vi "GESTIONE ALIMENTATORI.vi"(10 "Sub Panel alim1":refnum<vi>, 11 "Alimentatore":i32=1) -> ()   [LabVIEW 2019]
uses:
  TypeDef/Alimentatore.ctl
  Rampe e compensazioni/Comandi alimentatori.ctl
  TypeDef/Comandi_Alimentatore.ctl
  cDAQ_PLC Folder/cDAQ/SET SINGLE DO.ctl
  cDAQ_PLC Folder/cDAQ/DO List.ctl
  cDAQ_PLC Folder/cDAQ/SET SINGLE AO.ctl
  cDAQ_PLC Folder/cDAQ/AO List.ctl
  cDAQ_PLC Folder/cDAQ/SET ARRAY DO.ctl
  Stato alimentatore 1.vi
  Fine rampa sinus penta.vi
  Global_All_Data.vi
  Global FINE AVVIO.vi
  Global rapporto trasfo.vi
  Global dati targa SINUSPENTA.vi
panel:
  in  "Time Target (s)":dbl=1.0
  out "RPM":dbl
  out "Alimentatore selez":i32
  out "Iteration in Loop 1":i32
  out "Message":string
  in  "y 2":dbl=49.0 format="%#_13g"
  in  "y":dbl=5.0 format="%#_13g"
  out "Nome":string
  in  "SELEZIONA ALIMENTATORE":bool
  in  "indice alimentatore":i8
  out "Boolean":bool
  in  "Alimentatore":T1 {"Status ref"."RIF 2" scale=0.0..100.0; "Status ref"."RIF 1" scale=0.0..400.0}
  out "Alimentatore 1":T1 {"Status ref"."RIF 2" scale=0.0..100.0; "Status ref"."RIF 1" scale=0.0..100.0}
  in  "Salva alimentatori":bool
  in  "EXIT":bool
  out "EXIT":bool
  out "Comandi alimentatori":T2[](array[typedef])
  in  "Misure":T3
  in  "Array pannelli alimentatori":T4(array[cluster])
  in  "Array alimentatori":T5[](array[typedef]) {"Controllo Rif 2"."Precisione pid" format="%#_13g"; "Controllo Rif 2"."PID gains"."derivative time (Td, min)" format="%.3f"; "Controllo Rif 2"."PID gains"."integral time (Ti, min)" format="%.3f"; "Controllo Rif 2"."PID gains"."proportional gain (Kc)" format="%.3f"; "Controllo Rif 1"."Precisione pid" format="%#_13g"; "Controllo Rif 1"."PID gains"."derivative time (Td, min)" format="%.3f"; "Controllo Rif 1"."PID gains"."integral time (Ti, min)" format="%.3f"; "Controllo Rif 1"."PID gains"."proportional gain (Kc)" format="%.3f"}
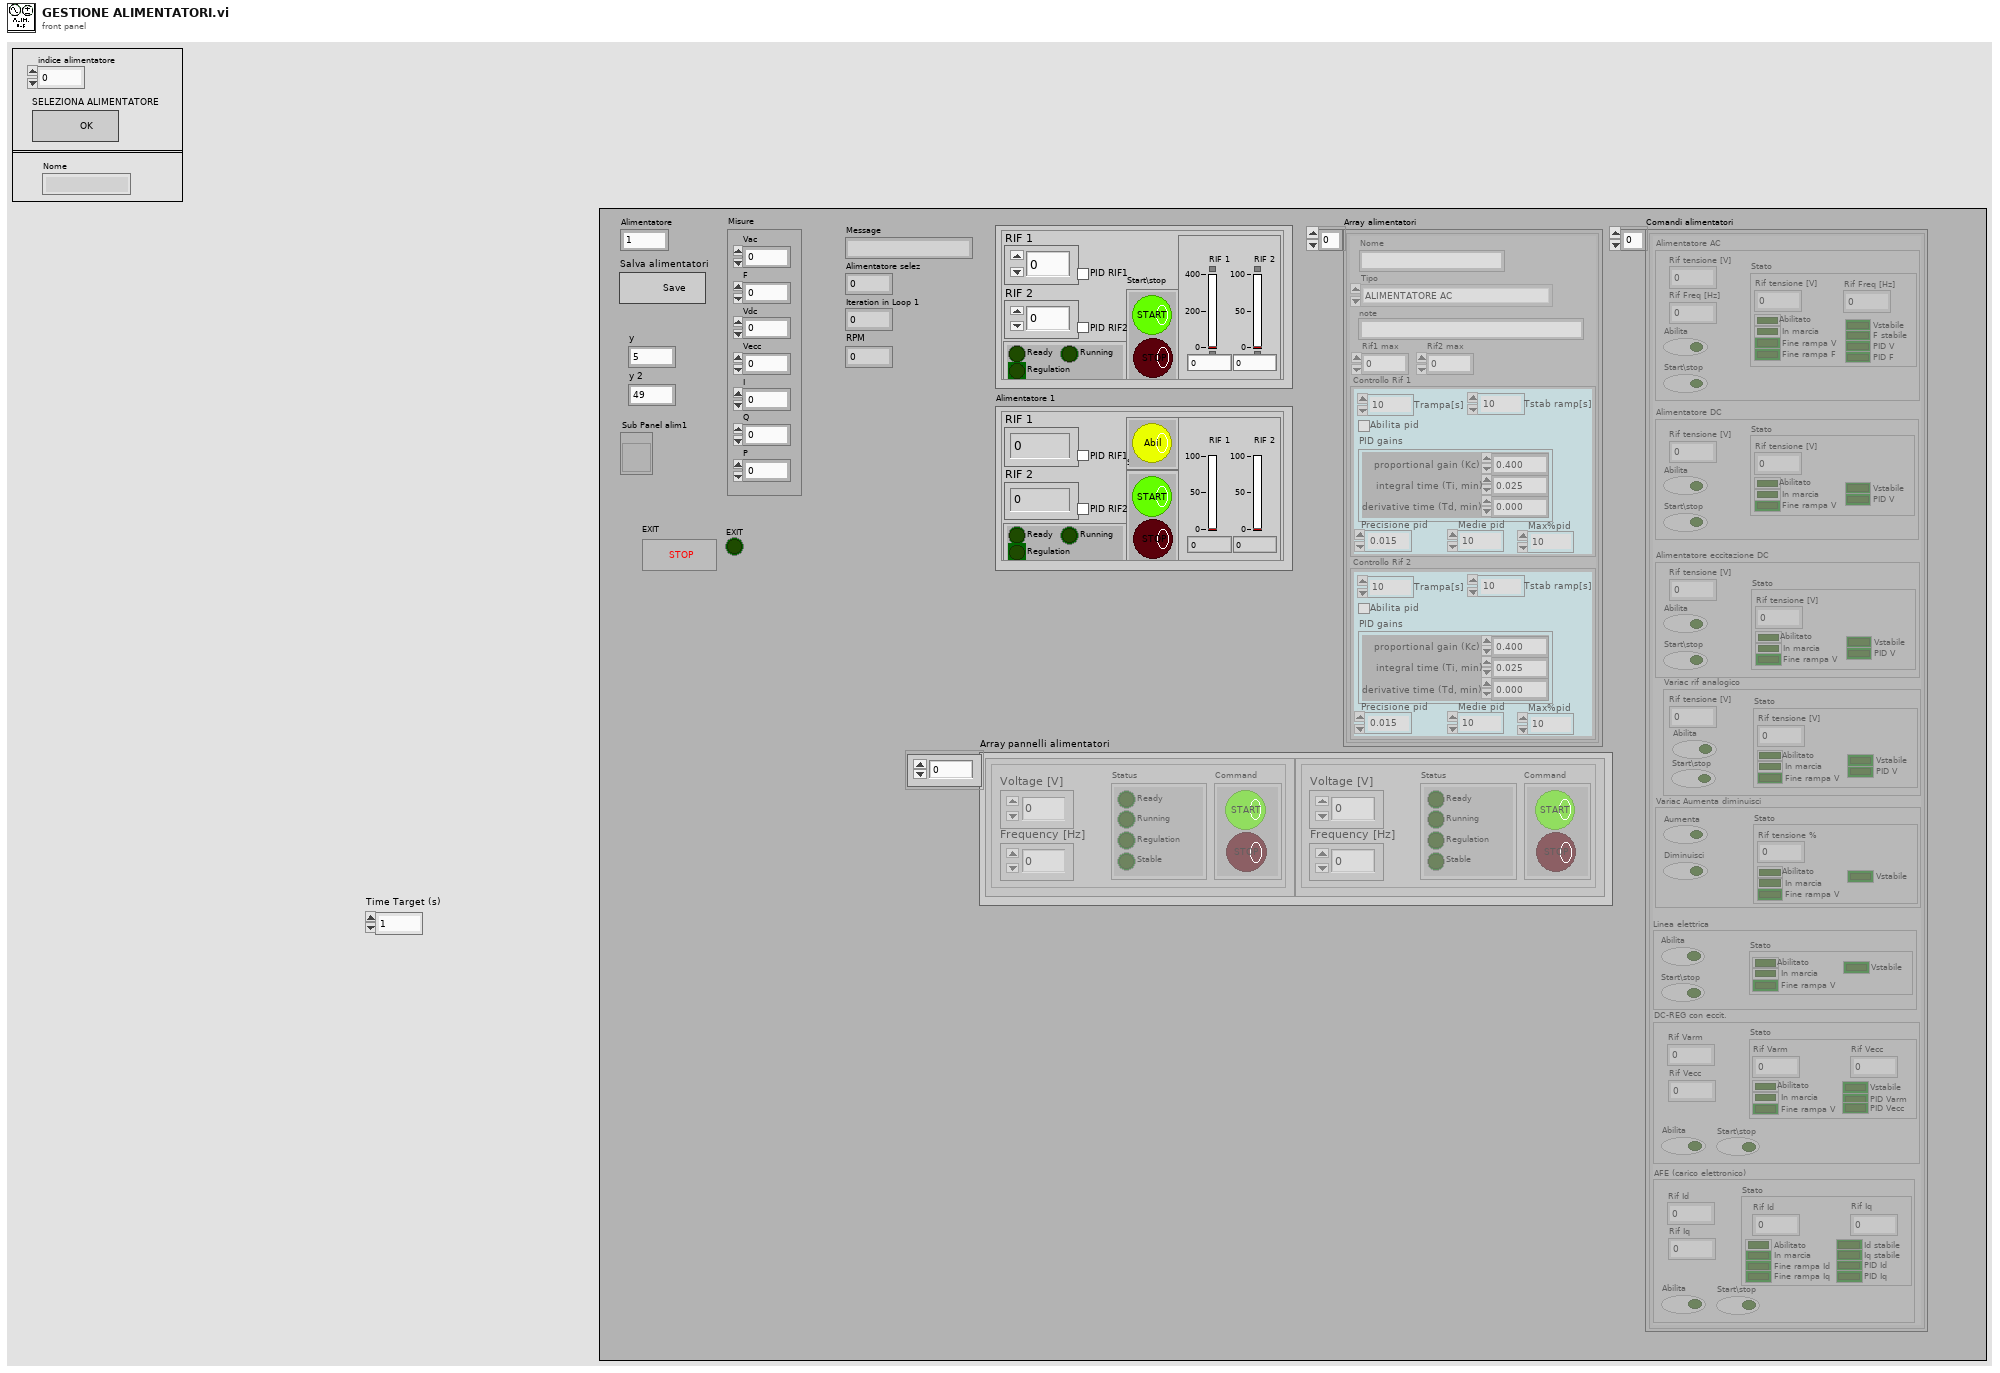
[diagram p1: front panel]
types:
  T1 = typedef "Comandi_Alimentatore.ctl" = cluster{"RIF 1":dbl, "RIF 2":dbl, "Status":cluster{"Ready":bool, "Running":bool, "Regulation":bool}, "Start\\stop":cluster{"Start":bool, "Stop":bool}, "PID RIF1":bool, "PID RIF2":bool, "Status ref":cluster{"RIF 1":dbl, "RIF 2":dbl}, "Abilita":cluster{"Abilita":bool}}
  T2 = typedef "Comandi alimentatori.ctl" = cluster{"Alimentatore AC":cluster{"Rif tensione [V]":dbl, "Rif Freq [Hz]":dbl, "Abilita":bool, "Start\\stop":bool, "Stato":cluster{"Rif tensione [V]":dbl, "Rif Freq [Hz]":dbl, "Abilitato":bool, "In marcia":bool, "Fine rampa V":bool, "Fine rampa F":bool, "Vstabile":bool, "F stabile":bool, "PID V":bool, "PID F":bool}}, "Alimentatore DC":cluster{"Rif tensione [V]":dbl, "Abilita":bool, "Start\\stop":bool, "Stato":cluster{"Rif tensione [V]":dbl, "Abilitato":bool, "In marcia":bool, "Fine rampa V":bool, "Vstabile":bool, "PID V":bool}}, "Variac rif analogico":cluster{"Rif tensione [V]":dbl, "Stato":cluster{"Rif tensione [V]":dbl, "Abilitato":bool, "In marcia":bool, "Fine rampa V":bool, "Vstabile":bool, "PID V":bool}, "Start\\stop":bool, "Abilita":bool}, "Variac Aumenta diminuisci":cluster{"Aumenta":bool, "Diminuisci":bool, "Stato":cluster{"Rif tensione %":dbl, "Abilitato":bool, "In marcia":bool, "Fine rampa V":bool, "Vstabile":bool}}, "Alimentatore eccitazione DC":cluster{"Rif tensione [V]":dbl, "Abilita":bool, "Start\\stop":bool, "Stato":cluster{"Rif tensione [V]":dbl, "Abilitato":bool, "In marcia":bool, "Fine rampa V":bool, "Vstabile":bool, "PID V":bool}}, "Linea elettrica":cluster{"Abilita":bool, "Start\\stop":bool, "Stato":cluster{"Abilitato":bool, "In marcia":bool, "Fine rampa V":bool, "Vstabile":bool}}, "DC-REG con eccit.":cluster{"Rif Varm":dbl, "Abilita":bool, "Start\\stop":bool, "Stato":cluster{"Rif Varm":dbl, "Abilitato":bool, "In marcia":bool, "Fine rampa V":bool, "Vstabile":bool, "PID Varm":bool, "Rif Vecc":dbl, "PID Vecc":bool}, "Rif Vecc":dbl}, "AFE (carico elettronico)":cluster{"Rif Id":dbl, "Abilita":bool, "Start\\stop":bool, "Stato":cluster{"Rif Id":dbl, "Rif Iq":dbl, "Abilitato":bool, "In marcia":bool, "Fine rampa Id":bool, "Fine rampa Iq":bool, "Id stabile":bool, "Iq stabile":bool, "PID Id":bool, "PID Iq":bool}, "Rif Iq":dbl}}
  T3 = cluster{"Vac":dbl, "F":dbl, "Vdc":dbl, "Vecc":dbl, "I":dbl, "Q":dbl, "P":dbl}
  T4 = cluster{"Voltage [V]":dbl, "Frequency [Hz]":dbl, "Status":cluster{"Ready":bool, "Running":bool, "Regulation":bool, "Stable":bool}, "Command":cluster{"Start":bool, "Stop":bool}}[]
  T5 = typedef "Alimentatore.ctl" = cluster{"Rif1 max":dbl, "Rif2 max":dbl, "Tipo":enum16{"ALIMENTATORE AC", "VARIAC AC rif analogico", "VARIAC AC aumenta diminuisci", "ALIMENTATORE DC", "ALIMENTATORE eccitazione DC", "LINEA ELETTRICA", "DCREG con eccitazione", "Carico elettronico AFE"}, "Nome":string, "Controllo Rif 1":cluster{"PID gains":cluster{"proportional gain (Kc)":dbl, "integral time (Ti, min)":dbl, "derivative time (Td, min)":dbl}, "Abilita pid":bool, "Precisione pid":dbl, "Medie pid":i32, "Trampa[s]":i32, "Tstab ramp[s]":i32, "Max%pid":i32}, "Controllo Rif 2":cluster{"PID gains":cluster{"proportional gain (Kc)":dbl, "integral time (Ti, min)":dbl, "derivative time (Td, min)":dbl}, "Abilita pid":bool, "Precisione pid":dbl, "Medie pid":i32, "Trampa[s]":i32, "Tstab ramp[s]":i32, "Max%pid":i32}, "note":string}
  T6 = cluster{"Message":string, "Message Data":variant}
  T7 = cluster{"RIF 1":dbl, "RIF 2":dbl, "Status":cluster{"Ready":bool, "Running":bool, "Regulation":bool, "Stable":bool}, "Command":cluster{"Start":bool, "Stop":bool}}
  T8 = enum16{"open", "replace", "create", "open or create", "replace or create", "replace or create with confirmation"}
  T9 = cluster{"RIF1":dbl, "RIF2":dbl, "Status":cluster{"Ready":bool, "Running":bool, "Regulation":bool, "Stable":bool}, "Command":cluster{"Start":bool, "Stop":bool}}[]
  T10 = cluster{"Voltage [V]":dbl, "Frequency [Hz]":dbl, "Status":cluster{"Ready":bool, "Running":bool, "Regulation":bool, "Stable":bool}, "Command":cluster{"Start":bool, "Stop":bool}}
  T11 = cluster{"RIF 1":dbl, "RIF 2":dbl, "Status":cluster{"Ready":bool, "Running":bool, "Regulation":bool, "Stable":bool}, "Command":cluster{"Start":bool, "Stop":bool}}[]
  T12 = cluster{"RIF1":dbl, "RIF2":dbl, "Status":cluster{"Ready":bool, "Running":bool, "Regulation":bool, "Stable":bool}, "Command":cluster{"Start":bool, "Stop":bool}}
  T13 = enum16{"ALIMENTATORE AC", "VARIAC AC rif analogico", "VARIAC AC aumenta diminuisci", "ALIMENTATORE DC", "ALIMENTATORE eccitazione DC", "LINEA ELETTRICA", "DCREG con eccitazione", "Carico elettronico AFE"}
  T14 = cluster{"PID gains":cluster{"proportional gain (Kc)":dbl, "integral time (Ti, min)":dbl, "derivative time (Td, min)":dbl}, "Abilita pid":bool, "Precisione pid":dbl, "Medie pid":i32, "Trampa[s]":i32, "Tstab ramp[s]":i32, "Max%pid":i32}
  T15 = cluster{"RIF 1":dbl, "RIF 2":dbl, "Abilitato":bool, "In marcia":bool, "Fine rampa RIF1":bool, "Fine rampa RIF2":bool, "Vstabile":bool, "F stabile":bool, "PID RIF1":bool, "PID RIF2":bool, "Alimentatore 1":T1}
  T16 = typedef "SET SINGLE DO.ctl" = cluster{"DO":T17, "Value":bool}
  T17 = typedef "DO List.ctl" = enum16{"OFF: ALL DO", "*ABILITA freno 1", "*ABILITA freno 2", "*ABILITA freno 3", "*START freno 1", "*START freno 2", "*START freno 3", "*STOP freno 1", "*STOP freno 3", "*STOP freno 2", "*Senso rot freno 1", "*Senso rot freno 2", "*Senso rot freno 3", "*Ctrl velocità freno 1", "*Ctrl velocità freno 2", "*Ctrl velocità freno 3", "*Ctrl coppia freno 1", "*Ctrl coppia freno 2", "*Ctrl coppia freno 3", "*ABILITA alimentatore 1", "*ABILITA alimentatore 2", "*ABILITA alimentatore 3", "*ABILITA alimentatore 4", "*START alimentatore 1", "*START alimentatore 2", "*START alimentatore 3", "*START alimentatore 4", "*STOP alimentatore 1", "*STOP alimentatore 2", "*STOP alimentatore 3", "*STOP alimentatore 4", "SENSO ROT alimentatore 1", "SENSO ROT alimentatore 2", "Abilita LEM 1000A", "Abilita LEM 300A", "Abilita sensori EXT WT", "B1 Seleziona linea 1", "B1 Seleziona linea 2", "B1 Seleziona linea 3", "B1 Seleziona linea 4", "B1 Seleziona linea 5", "B2 Seleziona linea 1", "B2 Seleziona linea 2", "B2 Seleziona linea 3", "B2 Seleziona linea 4", "B2 Seleziona linea 5", "*Reset allarmi", "*Start potenza AC", "*Stop potenza AC", "*Start potenza DC", "*Stop potenza DC", "*Start potenza DC eccit", "*Stop pontenza DC eccit", "Bypass res meter", "2nd canale res meter", "Enable res meter", "*Abilit teler ramo WT", "*Abil teler ramo princ Resit", "*Abil teler ramo 1 Resist", "*Abil teler ramo 2 Resist", "*Abil teler ramo 3 Resist", "*Abil cortocirc avvolgim", "*Controllo torsiometro B1", "*Controllo Torsiom B2", "*Scala torsiometro B1", "*Scala torsiometro B2", "*Collaudo in corso", "*Allarme presente", "Abilitazione elettroserratura", "Exit", "*Abilita collaudo", "*Abilita potenza trifase", "*Abilita potenza monofase", "*Abilita potenza DC", "*Abilita potenza DC eccit", "*Disabilita teleruttori potenza", "Set teleruttori prova a freddo", "Prova a freddo monofase", "Watchdog", "Forza DO PLC 3", "Forza DO PLC 2", "Forza DO PLC 1", "Forza DO cDAQ", "Scala 2000(T) 200(F) res meter", "Seleziona banco 1", "Seleziona banco 2", "Comando azionam in blocco", "Comando azionam reset", "Sensibilità freno 16 32 nm", "Reset Allarmi", "Carico res - Ramo 1", "Carico res - Ramo 2", "Carico res - Ramo 3", "Carico res - Ramo 4", "Carico res - Ramo 5", "Carico res - Ramo 6", "Carico res - Ramo 7", "Carico res - Ramo 8", "Carico res - Ramo 9", "Carico res - Ramo 10", "Carico res - Ramo 11", "Carico res - Start ventilatore", "Carico res - Stop ventilatore", "Abilita potenza solo freno", "Abilita AFE + freno trasc", "Abilita potenza carico resistivo", "Chiudi potenza AFE", "Apri potenza AFE", "Start AFE", "Config Banco2 TDE", "Misura diretto WT", "Ripristina centralina protezioni", "Abilita Scrittura Dati Keb", "Bench Selection(0-B1,1-B2)", "Select current mode", "Select torque mode", "Select speed mode", "Extenal alarm", "Enable Extenal program ", "Start ", "Stop", "Enable force mode", "Abilita linea 125 A", "Abilita linea 63 A", "Abilita linea 16 A", "Aum Tensione Variac", "Dim Tesnione Variac", "Abilita Ellecto Stractura", "Riprinto Emergenxe ", "Abilita Collaudo", "Disabilita Collaudo", "Abilita Ingresso Variac", "Abilita Uscita Variac", "Abilita ventilatore Variac"}
  T18 = typedef "SET SINGLE AO.ctl" = cluster{"AO":T19, "Value":dbl}
  T19 = typedef "AO List.ctl" = enum16{"OFF: ALL AO", "RIF VEL FRENO 1", "RIF VEL FRENO 2", "RIF VEL FRENO 3", "RIF COPPIA FRENO", "RIF COPPIA FRENO 1", "RIF COPPIA FRENO 2", "RIF COPPIA FRENO 3", "RIF CORRENTE FRENO 2", "RIF V ALIM 1", "RIF F ALIM 1", "RIF V ALIM 2", "RIF F ALIM 2", "RIF V ALIM 3", "RIF F ALIM 3", "RIF V ALIM 4", "RIF F ALIM 4", "FORZA AO PLC 3", "FORZA AO PLC 2", "FORZA AO PLC 1", "FORZA AO cDAQ", "Configura alimentatore keb", "Tempo rampa keb", "Condensatori", "Exit"}
  T20 = cluster{"Rif tensione [V]":dbl, "Rif Freq [Hz]":dbl, "Abilitato":bool, "In marcia":bool, "Fine rampa V":bool, "Fine rampa F":bool, "Vstabile":bool, "F stabile":bool, "PID V":bool, "PID F":bool, "Alimentatore 1":T1}
  T21 = typedef "SET ARRAY DO.ctl" = T16[]
  T22 = typedef "Cluster MISURE.ctl" = cluster{"MISURE NM":T23, "MISURE ALL":T24}
  T23 = typedef "MISURE NM.ctl" = cluster{"Banco":string, "Anno":string, "Numero":string, "Ntabella":string, "Misura":string, "Tipo Prova":string, "ProgressivoAcq":string, "Descrizione":string, "Data_ora":string, "t. acq [h:m:s]":string, "t. acq [min]":string, "t. acq [s]":string, "n [rpm]":string, "f [Hz]":string, "U1[V]":string, "U2 [V]":string, "U3 [V]":string, "U123_media [V]":string, "I1[A]":string, "I2[A]":string, "I3[A]":string, "I123_media [A]*I":string, "I_123_sbil [%]":string, "Ulin[V]":string, "Uc [V]":string, "Uaux [V]":string, "Ilin[A]*I":string, "Imar[A]":string, "Iaux[A]":string, "Uarm[V]":string, "Uecc[V]":string, "Iarm[A]*I":string, "Iecc[A]":string, "pf":string, "P1 [W]":string, "P1 [kW]":string, "Q [VAR]":string, "Q [kVAR]":string, "S [VA]":string, "S [kVA]":string, "P1arm[W]":string, "P1ecc[W]":string, "Parm[kW]":string, "P1ecc[kW]":string, "Cond[uF]":string, "P1_linea_6fili[W]":string, "P1_linea_6fili[kW]":string, "eta_gr_6fili [%]":string, "eta_inverter_6fili [%]":string, "pf_linea_6fili":string, "U4 [V]":string, "U5 [V]":string, "U6 [V]":string, "U456_media [V]":string, "I4 [A]":string, "I5 [A]":string, "I6 [A]":string, "I456_media [A]":string, "C [Nm]*C":string, "Cric [Nm]":string, "Cric\\Cnom":string, "Iric[A]":string, "Iric\\Inom":string, "P2_mecc [W]":string, "P2_mecc [kW]":string, "eta motore [%]":string, "Scorr[%]":string, "Tamb[°C]":string, "R1[ohm]":string, "R2[ohm]":string, "R3[ohm]":string, "Rmedia[ohm]":string, "DT_R1[°C]":string, "DT_R2[°C]":string, "DT_R3[°C]":string, "DT_media[°C]":string, "R_marcia[ohm]":string, "R_aux[ohm]":string, "DT_marcia[°C]":string, "DT_aux[°C]":string, "R_Arm[ohm]":string, "R_Ecc[ohm]":string, "DT_Arm[°C]":string, "DT_Ecc[°C]":string, "TambFreddo[°C]":string, "R1_freddo[ohm]":string, "R2_freddo[ohm]":string, "R3_freddo[ohm]":string, "Rmedia_freddo[ohm]":string, "R_Marcia_freddo[ohm]":string, "R_Aux_freddo[ohm]":string, "R_Arm_freddo[ohm]":string, "R_Ecc_freddo[ohm]":string, "TC1 [°C]":string, "TC2 [°C]":string, "TC3 [°C]":string, "TC4 [°C]":string, "TC5 [°C]":string, "TC6 [°C]":string, "TC7 [°C]":string, "TC8 [°C]":string, "PT1000_1[°C]":string, "PT1000_2[°C]":string, "PT1000_3[°C]":string, "Vdc eccitatrice[V]":string, "Idc eccitatrice[A]":string, "Vdc rotore[V]":string, "Idc rotore[A]":string, "Vac rotore[V]":string, "Iac rotore[V]":string, "V dinamo[V]":string, "Portata Q":string, "Pressione H":string, "U1'[V]":string, "U2'[V]":string, "U3'[V]":string, "I1'[A]":string, "I2'[A]":string, "I3'[A]":string, "U''R-N":string, "U''S-N":string, "U'' T-N":string, "U''R-S":string, "U''R-T":string, "U''S-T":string, "I1''[A]":string, "I2''[A]":string, "I3''[A]":string, "F''[Hz]":string, "P''[kW]":string, "CosFi''":string, "PT1000_4[°C]":string, "Scorta 3":string}
  T24 = typedef "Cluster misure ALL.ctl" = cluster{"Cluster READ NI":T25, "MISURE WT":T28, "Resistenze Resistomat":T29, "INTERFACCIA":T30, "FREDDO resistomat":cluster{"Res Ch1":dbl, "Res Ch2":dbl, "tAMB":dbl, "Res Ch3":dbl}, "STATO PLC 1":T35, "Res Ch2":dbl, "Res Ch2 2":dbl, "FREDDO res meter":cluster{"Res Ch1":dbl, "Res Ch2":dbl, "tAMB":dbl, "Res Ch3":dbl}, "Resistenze Res Meter":T29, "READ SINUS PENTA":T39, "STATO PLC 2":T40, "STATO PLC 3":T44, "DCREG":T48}
  T25 = typedef "Cluster NI.ctl" = cluster{"AI (0-10V)":cluster{"AI 0":dbl, "AI 1":dbl, "AI 2":dbl, "AI 3":dbl, "AI 4":dbl, "AI 5":dbl, "AI 6":dbl, "AI 7":dbl, "AI 8":dbl, "AI 9":dbl, "AI 10":dbl, "AI 11":dbl, "AI 12":dbl, "AI 13":dbl, "AI 14":dbl, "AI 15":dbl, "AI 16":dbl, "AI 17":dbl, "AI 18":dbl, "AI 19":dbl, "AI 20":dbl, "AI 21":dbl, "AI 22":dbl, "AI 23":dbl, "AI 24":dbl, "AI 25":dbl, "AI 26":dbl, "AI 27":dbl, "AI 28":dbl, "AI 29":dbl, "AI 30":dbl, "AI 31":dbl}, "StatoAO_Cdaq[0-10V]":cluster{"AO 1":dbl, "AO 2":dbl, "AO 3":dbl, "AO 4":dbl}, "Contatori [rpm]":cluster{"RPM 1":dbl, "RPM 2":dbl}, "StatoAO_Cdaq [4-20mA]":T26, "StatoDO_Cdaq":T27, "DI":cluster{"Scorta 0":bool, "Scorta 1":bool, "Scorta 2":bool, "Scorta 3":bool, "Scorta 4":bool, "Scorta 5":bool, "Scorta 6":bool, "Scorta 7":bool, "Scorta 8":bool, "Scorta 9":bool, "Scorta 10":bool, "Scorta 11":bool, "Scorta 12":bool, "Scorta 13":bool, "Scorta 14":bool, "Scorta 15":bool, "Scorta 16":bool, "Scorta 17":bool, "Scorta 18":bool, "Scorta 19":bool, "Scorta 20":bool, "Scorta 21":bool, "Scorta 22":bool, "Scorta 23":bool, "Scorta 24":bool, "Scorta 25":bool, "Scorta 26":bool, "Scorta 27":bool, "Scorta 28":bool, "Scorta 29":bool, "Scorta 30":bool, "Scorta 31":bool}, "AI (4-20mA)":cluster{"AI 0":dbl, "AI 1":dbl, "AI 2":dbl, "AI 3":dbl, "AI 4":dbl, "AI 5":dbl, "AI 6":dbl, "AI 7":dbl, "AI 8":dbl, "AI 9":dbl, "AI 10":dbl, "AI 11":dbl, "AI 12":dbl, "AI 13":dbl, "AI 14":dbl, "AI 15":dbl}, "TC [°C]":cluster{"tc 1":dbl, "tc 2":dbl, "tc 3":dbl, "tc 4":dbl}, "NI Read Values":cluster{"RPM":dbl, "Frequency":dbl, "Mod 1":cluster{"Torsiometro 1":dbl, "Torsiometro 2":dbl, "Strin Gauge 1":dbl, "Strin Gauge 2":dbl}, "Mod 2":cluster{"Termocoppia 1":dbl, "Termocoppia 2":dbl, "Termocoppia 3":dbl, "Termocoppia 4":dbl}, "Mod 3":cluster{"PT 100 1":dbl, "PT 100 2":dbl, "PT 100 3":dbl, "PT 100 4":dbl}}}
  T26 = typedef "StatoAO_cdaq.ctl" = cluster{"Cdaq_AO [0-10V] 0 for Torque":dbl, "Cdaq_AO [0-10V] 1":dbl, "Cdaq_AO [0-10V] 2":dbl, "Cdaq_AO [0-10V] 3":dbl}
  T27 = typedef "statoDO_Cdaq.ctl" = cluster{"Scorta 0":bool, "Scorta 1":bool, "Scorta 2":bool, "Scorta 3":bool, "Scorta 4":bool, "Scorta 5":bool, "Scorta 6":bool, "Scorta 7":bool, "Scorta 8":bool, "Scorta 9":bool, "Scorta 10":bool, "Scorta 11":bool, "Scorta 12":bool, "Scorta 13":bool, "Scorta 14":bool, "Scorta 15":bool, "Scorta 16":bool, "Scorta 17":bool, "Scorta 18":bool, "Scorta 19":bool, "Scorta 20":bool, "Scorta 21":bool, "Scorta 22":bool, "Scorta 23":bool, "Scorta 24":bool, "Scorta 25":bool, "Scorta 26":bool, "Scorta 27":bool, "Scorta 28":bool, "Scorta 29":bool, "Scorta 30":bool, "Scorta 31":bool}
  T28 = typedef "MISURE WT.ctl" = cluster{"URMS 1":dbl, "IRMS 1":dbl, "P 1":dbl, "S 1":dbl, "Q 1":dbl, "LAMBDA 1":dbl, "PHI 1":dbl, "F U 1":dbl, "F I 1":dbl, "NONE 1":dbl, "URMS 2":dbl, "IRMS 2":dbl, "P 2":dbl, "S 2":dbl, "Q 2":dbl, "LAMBDA 2":dbl, "PHI 2":dbl, "F U 2":dbl, "F I 2":dbl, "NONE 2":dbl, "URMS 3":dbl, "IRMS 3":dbl, "P 3":dbl, "S 3":dbl, "Q 3":dbl, "LAMBDA 3":dbl, "PHI 3":dbl, "F U 3":dbl, "F I 3":dbl, "NONE 3":dbl, "URMS SIGMA":dbl, "IRMS SIGMA":dbl, "P SIGMA":dbl, "S SIGMA":dbl, "Q SIGMA":dbl, "LAMBDA SIGMA":dbl, "PHI SIGMA":dbl, "F U SIGMA":dbl, "F I SIGMA":dbl, "NONE 4":dbl}
  T29 = typedef "ClusterRes.ctl" = cluster{"Res Ch1":dbl, "Res Ch2":dbl, "Res Ch3":dbl, "Tamb":dbl}
  T30 = typedef "INTERFACCIA.ctl" = cluster{"AI":cluster{"Portate":T31[], "Pressioni":T31[], "Coppie[Nm]":T31[], "Valvole prop %":T31[], "RPM":T31[], "Livelli":T31[], "Temperature":T31[], "Riferimenti %":T31[], "TENSIONI":T31[], "CORRENTI":T31[]}, "DI (logici)":cluster{"Start da pulsantiera":bool, "Stop da pulsantiera":bool, "Reset da pulsantiera":bool, "Sistema OK":bool, "Collaudo abilitato":bool, "Potenza trifase abilitata":bool, "Potenza monofase abilitata":bool, "Potenza DC abilitata":bool, "Potenza DC ECC abilitata":bool, "Start alimentazione AC":bool, "Start alimentazione DC":bool, "Start DC eccitazione":bool, "Teleruttore WT abilitato":bool, "Teleruttore Resistomat abilitato":bool, "Teleruttore corto fasi":bool, "Ramo 1 resistomat":bool, "Ramo 2 resistomat":bool, "Ramo 3 resistomat":bool, "B1 Scelta linea elettrica 1":bool, "B1 Scelta linea elettrica 2":bool, "B1 Scelta linea elettrica 3":bool, "B1 Scelta linea elettrica 4":bool, "B1 Scelta linea elettrica 5":bool, "B2 Scelta linea elettrica 1":bool, "B2 Scelta linea elettrica 2":bool, "B2 Scelta linea elettrica 3":bool, "B2 Scelta linea elettrica 4":bool, "B2 Scelta linea elettrica 5":bool, "Rotore bloccato 1":bool, "Rotore bloccato 2":bool, "FRENO 1 abilitato":bool, "FRENO 1 run":bool, "FRENO 1 senso rotaz":bool, "FRENO 1 ctrl velocità":bool, "FRENO 2 abilitato":bool, "FRENO 2 run":bool, "FRENO 2 senso rotaz":bool, "FRENO 2 ctrl velocità":bool, "ALIM 1 abilitato":bool, "ALIM 1 run":bool, "ALIM 2 abilitato":bool, "ALIM 2 run":bool, "ALIM 3 abilitato":bool, "ALIM 3 run":bool, "FRENO 1 ctrl coppia":bool, "FRENO 2 ctrl coppia":bool, "FRENO 3 ctrl coppia":bool, "DI (logici) aggiuntivi impianto":cluster{"Solo freno abilitato":bool, "Carico resistivo abilitato":bool, "AFE+freno abilitato":bool, "Protezioni chiuse":bool, "Start potenza AFE":bool, "AFE in marcia":bool}, "Misura corrente diretta WT":bool, "Misura corrente sens ext":bool, "Sens ext abilitati":bool}, "AO non scalati":T33, "AO scalati":T33, "DO (logici)":T34}
  T31 = typedef "ClusterMisura_e_Unità_INPUT.ctl" = cluster{"Misura":dbl, "UM":T32, "Descrizione":string}
  T32 = typedef "UnitàMisura.ctl" = enum16{"V", "mA", "Bar", "RPM", "m3/s", "m3/min", "m3/h", "l/s", "l/min", "in3/min", "ft3/min", "gpm", "igpm", "igph", "%", "°C", "m", "Nm", "A"}
  T33 = typedef "Lista AO sistema.ctl" = cluster{"FRENO1 rif vel":dbl, "FRENO1 rif Coppia":dbl, "FRENO2 rif vel":dbl, "FRENO2 rif Coppia":dbl, "ALIM1 rif V":dbl, "ALIM1 rif F":dbl, "ALIM2 rif V":dbl, "ALIM2 rif F":dbl, "ALIM3 rif V":dbl, "ALIM3 rif F":dbl, "Fnom keb":dbl, "Rpm nom keb":dbl, "Pnom keb":dbl, "Inom keb":dbl, "Vnom keb":dbl, "Rpm max keb":dbl, "Tempo rampa keb":dbl, "Tipo Mot keb":dbl, "FRENO  rif Coppia ":dbl, "FRENO  rif  Corrente":dbl}
  T34 = typedef "DOinterfaccia.ctl" = cluster{"Scelta banco 1":bool, "Scelta banco 2":bool, "Scelta banco 3":bool, "FRENO 1 abilita":bool, "FRENO 1 start":bool, "FRENO 1 senso rotaz":bool, "FRENO 1 ctrl velocità":bool, "FRENO 2 abilita":bool, "FRENO 2 start":bool, "FRENO 2 senso rotaz":bool, "FRENO 2 ctrl velocità":bool, "ALIM 1 abilita":bool, "ALIM 1 start":bool, "ALIM 2 abilita":bool, "ALIM 2 start":bool, "ALIM 3 abilita":bool, "ALIM 3 start":bool, "Abilita linea trifase":bool, "Abilita linea monofase":bool, "Abilita linea dc":bool, "Abilita linea dc eccit":bool, "B1 Linea elettrica 1":bool, "B1 Linea elettrica 2":bool, "B1 Linea elettrica 3":bool, "B1 Linea elettrica 4":bool, "B1 Linea elettrica 5":bool, "B2 Linea elettrica 1":bool, "B2 Linea elettrica 2":bool, "B2 Linea elettrica 3":bool, "B2 Linea elettrica 4":bool, "B2 Linea elettrica 5":bool, "Start potenza AC":bool, "Stop pontenza AC":bool, "Start potenza DC":bool, "Stop potenza DC":bool, "Start potenza eccitaz":bool, "Stop potenza eccitaz":bool, "Reset allarmi":bool, "watchdog":bool, "Scala torsiometro B1":bool, "Controllo torsiom B1":bool, "Scala torsiometro B2":bool, "Controllo torsiom B2":bool, "Teleruttore WT abilita":bool, "Teleruttore Resistomat abilita":bool, "Teleruttore corto fasi":bool, "Ramo 1 resistomat":bool, "Ramo 2 resistomat":bool, "Ramo 3 resistomat":bool, "Collaudo in corso":bool, "Allarme presente":bool, "Enable Res Meter":bool, "Bypass Res Meter":bool, "2nd canale Res Meter":bool, "Scala 200/2000 res meter":bool, "Taratura res meter":bool, "FRENO 1 ctrl coppia":bool, "FRENO 2 ctrl coppia":bool, "FRENO 3 ctrl coppia":bool, "Aggiuntivi impianto":cluster{"Senso rotazione alim 1":bool, "Senso rotazione alim 2":bool}, "ALIM 1 stop":bool, "ALIM 2 stop":bool, "ALIM 3 stop":bool, "FRENO 1 stop":bool, "FRENO 2 stop":bool, "FRENO 3 stop":bool, "B1 configurazione freno B":bool, "B2 configurazione freno B":bool, "Abilita scrittura KEB":bool, "Bench Selection (0-B1,1-B2)":bool, "Select current mode":bool, "Select torque mode":bool, "Select speed mode":bool, "Start":bool, "Stop":bool, "Block":bool, "Enable Force mode":bool, "Abilita linea 125 A":bool, "Abilita linea 63 A":bool, "Abilita linea 16 A":bool, "Aum Tensione Variac":bool, "Dim Tesnione Variac":bool, "Abilita ellectro stractura":bool, "Risprinito Emergence":bool, "Abilita collaudo":bool, "Disabilita collaudo":bool, "External Alaram":bool, "Enable external program":bool, "Reset":bool, "Abilita Ingresso Variac":bool, "Abilita Ventilatore Variac":bool, "Abilita Uscita Variac ":bool}
  T35 = typedef "STATO PLC 1.ctl" = cluster{"USCITE PLC":T36, "Stato DI_PLC":cluster{"Sistema OK":bool, "Rotore bloccato":bool, "Scorta 1":bool, "Prova diretto inverter":bool, "Prova con filtro LC":bool, "Teleruttore WT abilitato":bool, "Alim sinus penta abilitato":bool, "Alim sinus penta in marcia":bool, "Freno abilitato":bool, "Freno in marcia":bool, "Senso rotazione freno":bool, "Potenza abilitata":bool, "Scorta 3":bool, "Scorta 4":bool, "scorta 5":bool, "scorta 6":bool}, "AI plc":cluster{"Allarmi 1":dbl, "Allarmi 2":dbl, "Scorta 1":dbl, "Scorta 2":dbl, "RPM mot prova":dbl, "I mot prova":dbl, "RPM freno":dbl, "I freno":dbl, "Scorta 3":dbl, "Scorta 4":dbl}}
  T36 = typedef "Uscite PLC 1.ctl" = cluster{"AO (real) 2":cluster{"SCORTA 1":dbl, "SCORTA 2":dbl, "SCORTA 3":dbl, "SCORTA 4":dbl, "SCORTA 5":dbl, "SCORTA 6":dbl, "SCORTA 7":dbl, "SCORTA 8":dbl}, "statoAO_PLC out":T37, "DO (bit)":T38}
  T37 = typedef "statoAO_plc_1.ctl" = cluster{"Rif Lim coppia freno [%]":dbl, "Rif rpm freno [%]":dbl, "Rif coppia freno [%]":dbl, "Rif V alimentatore [%]":dbl, "Rif F alimentatore [%]":dbl}
  T38 = typedef "StatoDO_PLC_1.ctl" = cluster{"Scelta banco 1":bool, "Set dati motore freno 2":bool, "Diretto inverter":bool, "Filtro LC":bool, "Marcia ALIM (1s)":bool, "Marcia FRENO (1s)":bool, "Stop AFE (1s)":bool, "Stop freno (1s)":bool, "Reset allarmi":bool, "Watchdog":bool, "Senso rotazione":bool, "Abilita collaudo (1s)":bool, "Disabilita collaudo (1s)":bool, "Abilitazione ALIM":bool, "Abilitazione FRENO":bool, "Teleruttore WT":bool, "Senso rot motore prova":bool, "Scorta 7":bool, "Scorta 8":bool, "Scorta 9":bool, "Scorta 10":bool, "Scorta 11":bool, "Scorta 12":bool, "Scorta 13":bool}
  T39 = typedef "Parametri inverter letti.ctl" = cluster{"Menù Misure motore (M000-M030)":cluster{"Rif vel a regime (int)":u16, "Rif vel a regime (dec)":u16, "Rif vel dopo rampe (int)":u16, "Rif vel dopo rampe (dec)":u16, "RPM motore (int)":u16, "RPM motore (dec)":u16, "FREQout inverter":u16, "Rif coppia a regime(Nm)":u16, "Richiesta di coppia (Nm)":u16, "Coppia generata dal motore(Nm)":u16, "Rif coppia a regime(%)":u16, "Richiesta di coppia (%)":u16, "Coppia generata dal motore(%)":u16, "Coppia max richiesta prima delle rampe(Nm)":u16, "Coppia max richiesta dopo le rampe(Nm)":u16, "Limite di velocità prima delle rampe":u16, "Limite di velocità dopo le rampe":u16, "Coppia max richiesta prima delle rampe(%)":u16, "Coppia max richiesta dopo le rampe(%)":u16, "Rif di flusso":u16, "Corrente di uscita":u16, "Capacità termica del motore":u16, "Tensione di uscita":u16, "Potenza di uscita":u16, "Energia consumata (LSword)":u16, "Energia consumata (MSword)":u16, "Tensione bus DC":u16, "Tensione di rete":u16}, "Menù regolatore PID (M018-M024)":cluster{"Rif PID a regime(%)":u16, "Rif pid dopo rampe(%)":u16, "Retroazione del pid(%)":u16, "Errore del pid(%)":u16, "uscita del pid(%)":u16, "Rif del pid dopo le rampe":u16, "Retroazione del pid":u16}, "Menù ingressi digitali (M031-M036)":cluster{"Ingressi digitali ritardati":u16, "Ingressi digitali istantanei":u16, "Moresettiera comando loc":u16, "Morsett comando da seriale":u16, "Morsett comando bus di campo":u16, "Ing dig ausiliari da morsettiera":u16, "Ing dig ausiliari da seriale":u16}, "Menù riferimenti (M037-M051)":cluster{"Rif analog est REF":u16, "Rif analog est AIN1":u16, "Rif analog est AIN2":u16, "Rif analog est XAIN4":u16, "Rif analog est XAIN5":u16, "Rif velocità da seriale(int)":u16, "Rif velocità bus di campo(int)":u16, "Rif coppia da seriale":u16, "Rif coppia bus di campo":u16, "Rif del PID da seriale":u16, "Rif del PID da bus di campo":u16, "Retroazione del PID da seriale":u16, "Retroazione del PIDda bus di campo":u16, "Rif da encoder":u16, "Rif in frequenza":u16, "Rif velocità da seriale(dec)":u16, "Rif velocità bus di campo(dec)":u16}, "Menù rampe (P009-P033)":cluster{"Tempo di dec rampa di vel 1":u16, "Tempo di acc rampa di vel 2":u16, "Tempo di dec rampa di vel 2":u16, "Tempo di acc rampa di vel 1":u16, "Unità di mis tempi rampe vel 1/2":u16, "Tempo di acc rampa di vel 3":u16, "Tempo di dec rampa di vel 3":u16, "Tempo di acc rampa di vel 4":u16, "Tempo di dec rampa di vel 4":u16, "Unità di mis tempi rampe vel 3/4":u16, "Selettore arrottondam rampe":u16, "Tempo di arrotond iniz rampa acc":u16, "Tempo di arrotond finale rampa acc":u16, "Tempo di arrotond iniz rampa dec":u16, "Tempo di rampa di salita rif coppia":u16, "Tempo di rampa di discesa rif coppia":u16, "Unità di misura rampa coppia":u16, "Tempo rampa acc marcia jog":u16, "Tempo rampa dec marcia jog":u16, "Reset acc ai cambi pendenza":u16, "rampa di acc in fire mode":u16, "rampa di dec in fire mode":u16, "Tempo di arrotond finale rampa dec":u16}, "Menù controllo motore(C008-C128)":cluster{"Numero motori configurati":u16, "Tipo algoritmo di controllo Mot1":u16, "Tipo rif Mot1":u16, "Tensione nominale rete":u16, "Retroaz di vel da encoder Mot1":u16, "Tipo curva V/f Mot1":u16, "Rotazione delle fasi Mot1":u16, "Freq nominale del motore Mot1":u16, "RPM nominali del motore Mot1":u16, "Potenza nominale del motore Mot1":u16, "Corrente nominale del motore Mot1":u16, "Tensione nominale del motore mot1":u16, "Potenza a vuoto del motore Mot1":u16, "Corrente a vuoto del motore Mot1":u16, "Resistenza statorica del motore Mot1":u16, "Induttanza di dispersione Mot1":u16, "Induttanza mutua motore":u16, "Costante di tempo rotorica":u16, "Costante di tempo filtro pb":u16, "Velocità minima motore":u16, "Velocità massima motore":u16}, "Menù configurazione PID":cluster{"Selezione riferimento n.1":u16, "Selezione retroazione n.1":u16, "Modalità di fuzionamento PID":u16, "Termine derivativo calcolato su err o mis":u16, "Proporz moltiplica deriv e integrale":u16, "Azione del PID":u16}, "ID":dbl, "Menù uscite digitali":cluster{"MDO4 Inverter pronto":u16}, "Fcarrier":cluster{"Fcarrier Min (Hz)":u16, "Fcarrier Max (Hz)":u16}, "stato inverter M089":dbl, "Riferimenti":cluster{"Rif tensione":u16, "Rif velocità":u16}, "Comunicazione":bool, "Modalità stop":dbl}
  T40 = typedef "STATO PLC 2.ctl" = cluster{"USCITE PLC":T41, "Stato DI_PLC":cluster{"Sistema ok":bool, "Relè Resistomat abilitato":bool, "Freno abilitato":bool, "Freno in marcia":bool, "scorta b":bool, "scorta a":bool, "scorta 1":bool, "scorta 2":bool, "scorta 3":bool, "scorta 4":bool, "Scorta 5":bool, "Scorta 6":bool, "Scorta 7":bool, "Scorta 8":bool, "Scorta 9":bool, "Scorta 10":bool}, "AI plc":cluster{"Allarmi 1":dbl, "Allarmi 2":dbl, "TC 1":dbl, "TC 2":dbl, "TC 3":dbl, "TC 4":dbl, "TC 5":dbl, "TC 6":dbl, "TC 7":dbl, "TC 8":dbl, "PT1000 1":dbl, "PT1000 2":dbl, "PT1000 3":dbl, "PT1000 4":dbl}}
  T41 = typedef "Uscite PLC 2.ctl" = cluster{"AO (real) 2":cluster{"SCORTA 1":dbl, "SCORTA 2":dbl, "SCORTA 3":dbl, "SCORTA 4":dbl, "SCORTA 5":dbl, "SCORTA 6":dbl, "SCORTA 7":dbl, "SCORTA 8":dbl}, "statoAO_PLC out":T42, "DO (bit)":T43}
  T42 = typedef "statoAO_plc_2.ctl" = cluster{"Condensatori":dbl, "Scorta 1":dbl, "Scorta 2":dbl}
  T43 = typedef "StatoDO_PLC_2.ctl" = cluster{"Relè misura resistomat":bool, "Misura res ramo 1":bool, "Misura res ramo 2":bool, "Misura res ramo 3":bool, "Scelta banco 2":bool, "Scala Torsiometro":bool, "Ctrl torsiometro":bool, "Select current mode":bool, "Select Torque mode":bool, "Select speed mode":bool, "Watchdog":bool, "Scorta":bool, "Scorta 2":bool, "Scorta 3":bool, "Scorta 4":bool, "Scorta 5":bool, "Bench selection":bool, "External alarm":bool, "Enable external program":bool, "Reset allarmi":bool, "Start":bool, "Stop":bool, "Block":bool, "Scorta 6":bool}
  T44 = typedef "STATO PLC 3.ctl" = cluster{"USCITE PLC":T45, "Stato DI_PLC":cluster{"Sistema OK":bool, "Rotore bloccato":bool, "Filtro LC":bool, "Bypass Filtro LC":bool, "Scelta Trasformatore":bool, "Scelta Bypass trasformatore":bool, "Teleruttore wt abilitato":bool, "Alimentatore abilitato":bool, "Alimentatore in marcia":bool, "Scorta 1":bool, "Scorta 2":bool, "Scorta 3":bool, "Potenza abilitata":bool, "Alimentatore in allarme":bool, "Scorta 4":bool, "Conferma dati KEB":bool, "Scorta 5":bool, "Warning Inverter Alimentatore":bool, "Variac Abilitato":bool, "Linea 125 A abilitata":bool, "Linea 63 A abilitata":bool, "Linea 16 A abilitata":bool, "Scorta 6":bool, "Enable force mode":bool}, "AI plc":cluster{"Allarmi 1":dbl, "Allarmi 2":dbl, "RPM motore prova":dbl, "Corrente motore prova":dbl, "RPM freno":dbl, "Corrente freno":dbl, "Tipo motore keb":dbl, "I nom keb":dbl, "RPM nom keb":dbl, "V nom keb":dbl, "F nom keb":dbl, "T rampa keb":dbl, "scorta":dbl, "Scorta 2":dbl}}
  T45 = typedef "Uscite PLC 3.ctl" = cluster{"AO (real) 2":cluster{"SCORTA 1":dbl, "SCORTA 2":dbl, "SCORTA 3":dbl, "SCORTA 4":dbl, "SCORTA 5":dbl, "SCORTA 6":dbl, "SCORTA 7":dbl, "SCORTA 8":dbl}, "statoAO_PLC out":T46, "DO (bit)":T47}
  T46 = typedef "statoAO_plc_3.ctl" = cluster{"Rif velocità alimentatore":dbl, "Scorta":dbl, "Tipo Motore  keb":dbl, "I nom keb":dbl, "RPM nom keb":dbl, "V nom keb":dbl, "F nom keb":dbl, "t rampa keb":dbl}
  T47 = typedef "StatoDO_PLC_3.ctl" = cluster{"Select linea Inverter":bool, "Abilita sense wattmetro":bool, "Bypass filtro LC":bool, "Filtro LC":bool, "Bypass trasformatore":bool, "Trasformatore":bool, "Abilita uscite variac":bool, "Abilita linea 125 A":bool, "Abilita linea 63 A":bool, "Abilita linea 16 A":bool, "Abilita Scrittura Dati Keb":bool, "Abilita alimentatore":bool, "Marcia alimentatore (1s)":bool, "Stop alimentatore (1s)":bool, "Senso rot mot prova":bool, "Watchdog":bool, "Aumenta tensione variac":bool, "Diminuisci tensione variac ":bool, "Blocco elettroserrature":bool, "Ripristino emergence":bool, "Abilita ingresso variac":bool, "Abilita ventilatore variac":bool, "Reset Allarm":bool, "Scorta 1":bool, "Scorta 2":bool, "Scorta 3":bool, "Scorta 4":bool, "Scorta 5":bool, "Scorta 6":bool, "Scorta 7":bool, "Scorta 8":bool, "Scorta 9":bool, "Abilita collaudo":bool, "Disabilita collaudo ":bool, "Scorta 10":bool, "Scorta 11":bool, "Scorta 12":bool, "Scorta 13":bool, "Scorta 14":bool, "Scorta 15":bool}
  T48 = typedef "Parametri DCREG letti.ctl" = cluster{"Parametri di misura":cluster{"M000":dbl, "M001":dbl, "M002":dbl, "M003":dbl, "M004":dbl, "M005":dbl, "M006":dbl, "M007":dbl, "M008":dbl, "M009":dbl, "M010":dbl, "M011":dbl, "M012":dbl, "M013":dbl, "M014":dbl, "M015":dbl, "M016":dbl, "M017":dbl, "M018":dbl, "M019":dbl, "M020":dbl, "M021":dbl, "M022":dbl, "M023":dbl, "M024":dbl, "M025":dbl, "M026":dbl, "M027":dbl, "M028":dbl, "M029":dbl, "M030":dbl, "M031":dbl}, "Parametri di programmazione":cluster{"P000":dbl, "P001":dbl, "P002":dbl, "P003":dbl, "P004":dbl, "P005":dbl, "P006":dbl, "P010":dbl, "P011":dbl, "P012":dbl, "P013":dbl, "P014":dbl, "P015":dbl, "P016":dbl, "P030":dbl, "P031":dbl, "P032":dbl, "P033":dbl, "P034":dbl, "P035":dbl, "P036":dbl, "P037":dbl, "P038":dbl, "P039":dbl, "P040":dbl, "P050":dbl, "P051":dbl, "P052":dbl, "P053":dbl, "P054":dbl, "P055":dbl, "P056":dbl, "P057":dbl, "P058":dbl, "P059":dbl, "P060":dbl, "P061":dbl, "P062":dbl, "P070":dbl, "P071":dbl, "P073":dbl, "P074":dbl, "P076":dbl, "P077":dbl, "P079":dbl, "P080":dbl, "P082":dbl, "P083":dbl, "P084":dbl, "P085":dbl, "P086":dbl, "P087":dbl, "P088":dbl, "P100":dbl, "P101":dbl, "P102":dbl, "P103":dbl, "P104":dbl, "P110":dbl, "P111":dbl, "P120":dbl, "P121":dbl, "P122":dbl, "P123":dbl, "P124":dbl, "P125":dbl, "P126":dbl, "P127":dbl, "P128":dbl, "P129":dbl, "P130":dbl, "P131":dbl, "P132":dbl, "P133":dbl, "P134":dbl, "P150":dbl, "P151":dbl, "P152":dbl, "P153":dbl, "P154":dbl, "P155":dbl, "P156":dbl, "P157":dbl, "P158":dbl, "P170":dbl, "P171":dbl, "P172":dbl, "P173":dbl, "P174":dbl, "P175":dbl, "P176":dbl, "P177":dbl, "P178":dbl, "P179":dbl, "P180":dbl, "P181":dbl, "P182":dbl, "P183":dbl, "P184":dbl, "P185":dbl, "P186":dbl, "P187":dbl, "P188":dbl, "P189":dbl, "P190":dbl, "P191":dbl, "P192":dbl, "P193":dbl, "P194":dbl, "P195":dbl, "P196":dbl, "P197":dbl, "P198":dbl, "P199":dbl, "P211":dbl, "P212":dbl, "P213":dbl, "P214":dbl, "P215":dbl, "P216":dbl, "P217":dbl, "P221":dbl, "P222":dbl, "P223":dbl, "P224":dbl, "P230":dbl, "P231":dbl, "P240":dbl, "P250":dbl, "P251":dbl}, "Parametri di configurazione":cluster{"C000":dbl, "C001":dbl, "C002":dbl, "C010":dbl, "C011":dbl, "C012":dbl, "C014":dbl, "C015":dbl, "C016":dbl, "C017":dbl, "C018":dbl, "C030":dbl, "C050":dbl, "C051":dbl, "C052":dbl, "C060":dbl, "C061":dbl, "C062":dbl, "C063":dbl, "C070":dbl, "C072":dbl, "C074":dbl, "C090":dbl, "C091":dbl, "C092":dbl, "C093":dbl, "C094":dbl, "C100":dbl, "C101":dbl, "C102":dbl, "C103":dbl, "C105":dbl, "C106":dbl, "C107":dbl, "C108":dbl, "C110":dbl, "C111":dbl, "C112":dbl, "C120":dbl, "C121":dbl, "C122":dbl, "C130":dbl, "C131":dbl, "C132":dbl, "C133":dbl, "C134":dbl, "C135":dbl, "C141":dbl, "C142":dbl, "C143":dbl, "C150":dbl, "C151":dbl, "C153":dbl, "C154":dbl, "C155":dbl, "C156":dbl, "C157":dbl, "C158":dbl, "C159":dbl, "C160":dbl, "C161":dbl, "C162":dbl, "C163":dbl, "C164":dbl, "C165":dbl, "C170":dbl}, "Codice allarme":dbl, "Comunicazione":bool}
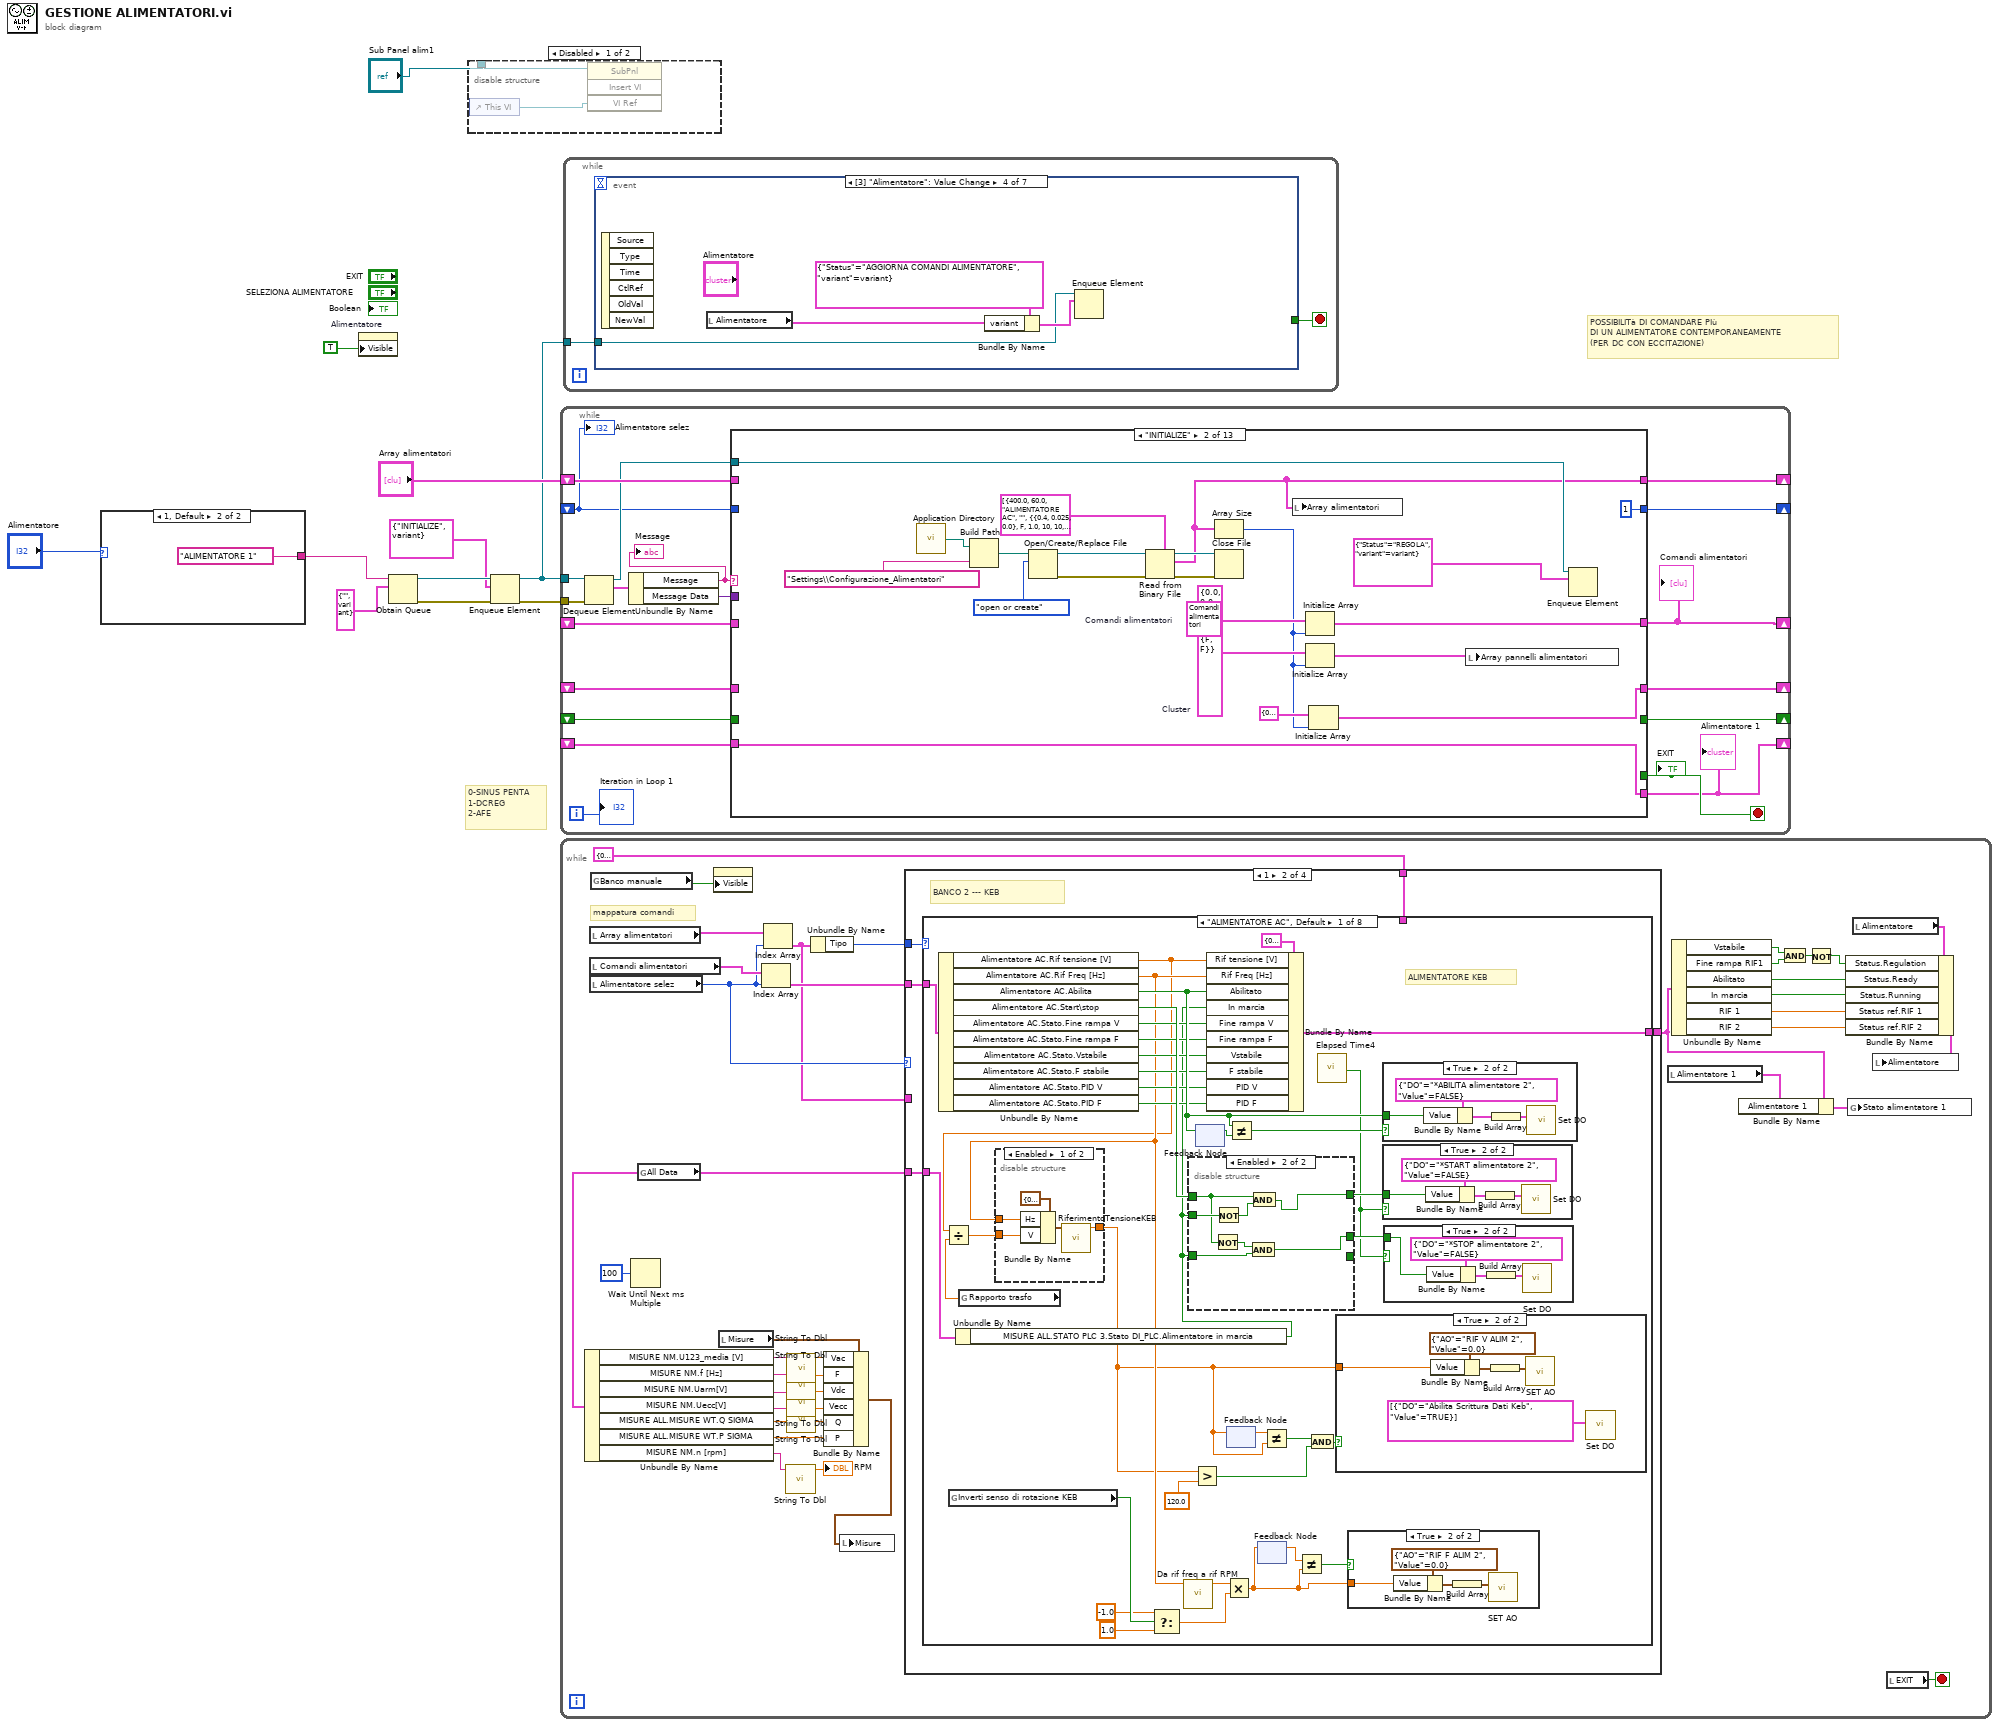
[diagram p0: block diagram]
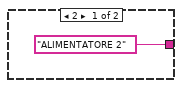
[diagram p3: hidden frame]
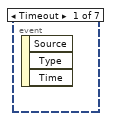
[diagram p4: hidden frame]
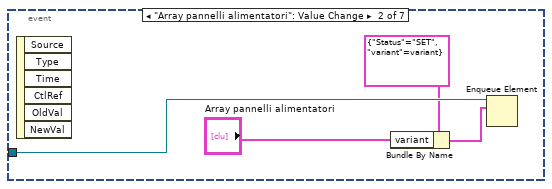
[diagram p5: hidden frame]
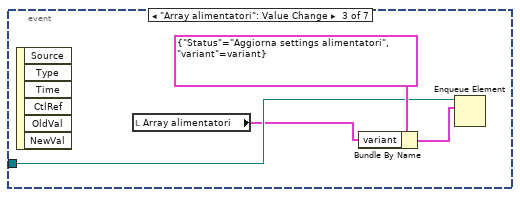
[diagram p6: hidden frame]
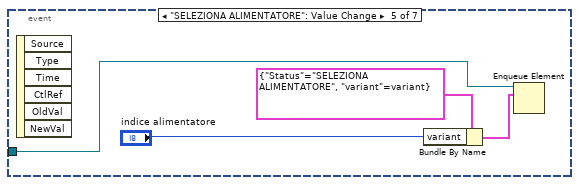
[diagram p7: hidden frame]
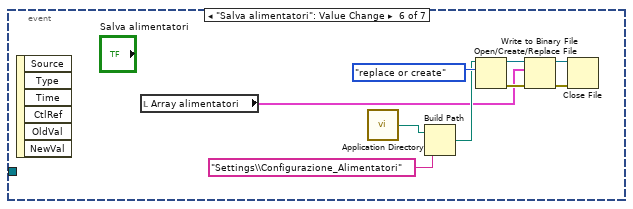
[diagram p8: hidden frame]
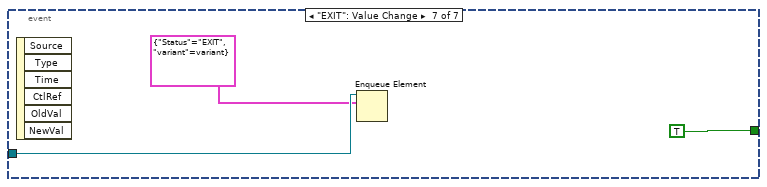
[diagram p9: hidden frame]
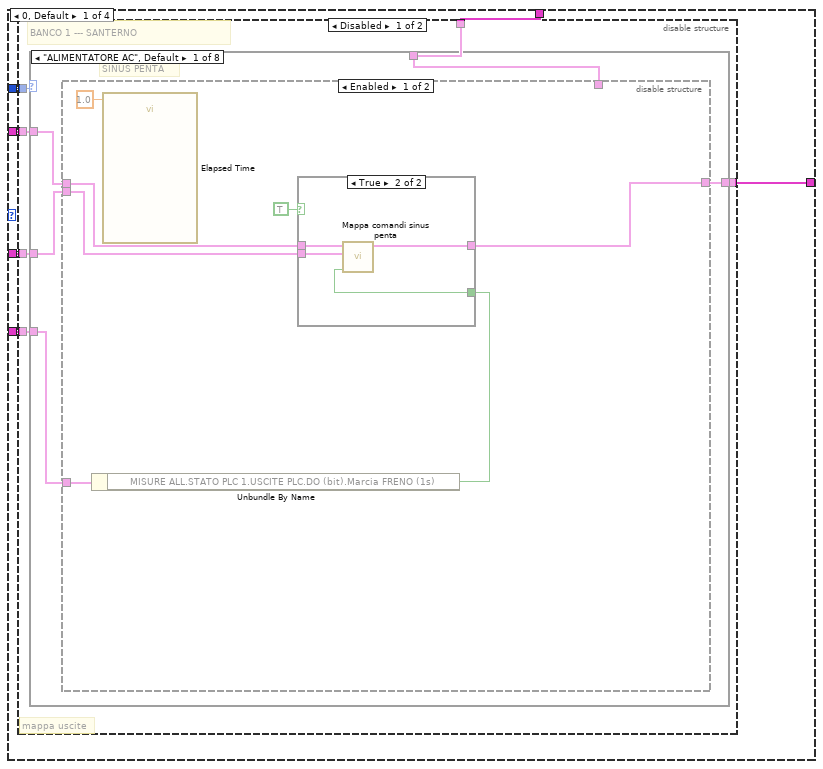
[diagram p10: hidden frame]
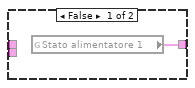
[diagram p11: hidden frame]
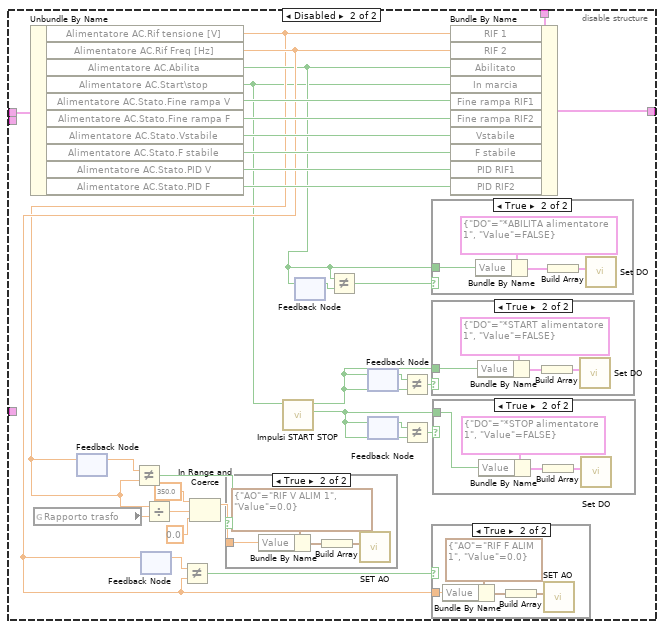
[diagram p12: hidden frame]
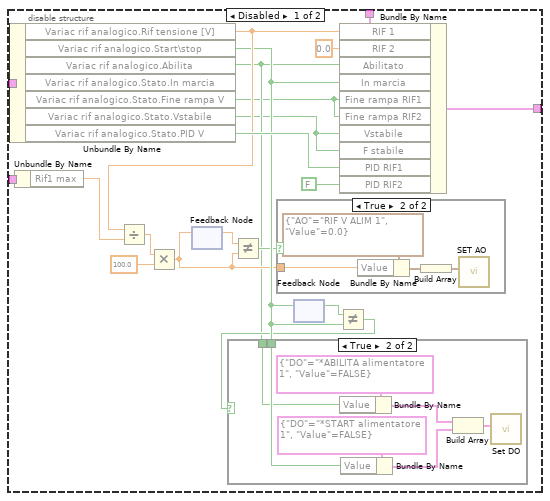
[diagram p19: hidden frame]
diagram:
  # "0-SINUS PENTA\n1-DCREG\n2-AFE"
  # "POSSIBILITà DI COMANDARE PIù\nDI UN ALIMENTATORE CONTEMPORANEAMENTE\n(PER DC CON ECCITAZIONE)"
  n1 = case shown="1, Default" "Alimentatore" {
    tunnel: ["ALIMENTATORE 2" ("name (unnamed)") "ALIMENTATORE 1" ("name (unnamed)")] -> w9
    frame 2 {
    }
    frame 1, Default {
    }
  }
  n2 = property on="Alimentatore" class="Clust (strict)"("Visible"=TRUE) -> ()  [unwired: 2 in, 2 out]
  n3 = Obtain Queue(name (unnamed)=w9, element data type=T6 {"Message"="", "Message Data"=variant} ("Message Cluster")) -> (queue out=w10:refnum<queue>, error out=w11:errorcluster)  [unwired: 3 in, 1 out]
  n4 = disable-structure shown="Disabled" {
    disable-tunnel: "Sub Panel alim1" -> [w15 _]
    frame Disabled {
      n5 = control-ref of="This VI"() -> (w14:refnum<vi>)
      n6 = invoke class="SubPnl" method="Insert VI"(reference=w15, "VI Ref"=w14) -> ()  [unwired: 2 in, 4 out]
    }
    frame Enabled {
    }
  }
  n7 = Enqueue Element(queue=w10, element=cluster{"Status":string, "variant":variant} {"Status"="INITIALIZE", "variant"=variant}, error in (no error)=w11) -> (queue out=w4:refnum<queue>, error out=w5:errorcluster)  [unwired: 1 in, 1 out]
  n8 = while {
    tunnel: w4 -> [w34]
    shift-right: [w30] -> _
    shift-left: "Array alimentatori" -> [w31]
    tunnel: w5 -> [w29]
    shift-right: [w17] -> _
    shift-left: _ -> [w28]
    shift-right: [w26] -> _
    shift-left: _ -> [w25]
    shift-right: [w24] -> _
    shift-left: _ -> [w23]
    shift-right: [w20] -> _
    shift-left: _ -> [w19]
    shift-right: [w16] -> _
    shift-left: _ -> [w18]
    i -> [w21]
    stop <- w27 stop-if-true
    n9 = Dequeue Element(queue=w34, error in (no error)=w29) -> (queue out=w22:refnum<queue>, element=w35:T6)  [unwired: 1 in, 2 out]
    n10 = Unbundle By Name(w35) -> ("Message"=w33:string, "Message Data"=w32:variant)
    "Message" <- w33
    n11 = case shown="\"INITIALIZE\"" w33 {
      tunnel: w32 -> [_ _ w84 w100 _ _ w286 w300 _ _ _ _ _]
      tunnel: w31 -> [w40 _ w81 w97 w105 w109 _ w297 w308 w342 w376 w408 w438]
      tunnel: [w40 w46 w79 w97 w105 w109 w284 w297 w308 w342 w376 w408 w438] -> w30
      tunnel: [w39 w60 w65 w96 w104 w123 w290 w296 w310 w344 w378 w410 w437] -> w17
      tunnel: w28 -> [w39 _ w65 w96 w104 w124 w290 w296 w312 w346 w380 w412 w437]
      tunnel: [_ _ _ _ _ _ _ _ _ _ _ _ w433] -> w27
      tunnel: [w38 w43 w73 w95 w103 w120 w289 w295 w309 w343 w377 w409 w436] -> w26
      tunnel: w25 -> [w38 _ w74 w95 w103 w120 w289 _ w309 w343 w377 w409 w436]
      tunnel: [_ _ TRUE w93 _ FALSE _ TRUE w311 w345 w379 w411 _] -> w24
      tunnel: w23 -> [_ _ _ w93 _ w121 _ _ w311 w345 w379 w411 _]
      tunnel: w22 -> [_ w59 w66 _ _ w118 _ w293 _ _ _ _ _]
      tunnel: [w36 w42 w63 w94 w101 w108 w288 w291 w302 w336 w370 w402 w434] -> w20
      tunnel: w19 -> [w36 w42 _ w94 w101 w108 w288 w291 w302 w336 w370 w402 w434]
      tunnel: [w37 1 w64 w98 w102 w111 w287 w292 w303 w337 w371 w403 w435] -> w16
      tunnel: w18 -> [w37 _ w64 _ w102 w111 w287 w292 w303 w337 w371 w403 w435]
      frame "False", Default {
      }
      frame "INITIALIZE" {
        w57 = T10 {"Voltage [V]"=0.0, "Frequency [Hz]"=0.0, "Status"={"Ready"=FALSE, "Running"=FALSE, "Regulation"=FALSE, "Stable"=FALSE}, "Command"={"Start"=FALSE, "Stop"=FALSE}}  # Cluster
        w61 = T2 {"Alimentatore AC"={"Rif tensione [V]"=0.0, "Rif Freq [Hz]"=0.0, "Abilita"=FALSE, "Start\\stop"=FALSE, "Stato"={"Rif tensione [V]"=0.0, "Rif Freq [Hz]"=0.0, "Abilitato"=FALSE, "In marcia"=FALSE, "Fine rampa V"=FALSE, "Fine rampa F"=FALSE, "Vstabile"=FALSE, "F stabile"=FALSE, "PID V"=FALSE, "PID F"=FALSE}}, "Alimentatore DC"={"Rif tensione [V]"=0.0, "Abilita"=FALSE, "Start\\stop"=FALSE, "Stato"={"Rif tensione [V]"=0.0, "Abilitato"=FALSE, "In marcia"=FALSE, "Fine rampa V"=FALSE, "Vstabile"=FALSE, "PID V"=FALSE}}, "Variac rif analogico"={"Rif tensione [V]"=0.0, "Stato"={"Rif tensione [V]"=0.0, "Abilitato"=FALSE, "In marcia"=FALSE, "Fine rampa V"=FALSE, "Vstabile"=FALSE, "PID V"=FALSE}, "Start\\stop"=FALSE, "Abilita"=FALSE}, "Variac Aumenta diminuisci"={"Aumenta"=FALSE, "Diminuisci"=FALSE, "Stato"={"Rif tensione %"=0.0, "Abilitato"=FALSE, "In marcia"=FALSE, "Fine rampa V"=FALSE, "Vstabile"=FALSE}}, "Alimentatore eccitazione DC"={"Rif tensione [V]"=0.0, "Abilita"=FALSE, "Start\\stop"=FALSE, "Stato"={"Rif tensione [V]"=0.0, "Abilitato"=FALSE, "In marcia"=FALSE, "Fine rampa V"=FALSE, "Vstabile"=FALSE, "PID V"=FALSE}}, "Linea elettrica"={"Abilita"=FALSE, "Start\\stop"=FALSE, "Stato"={"Abilitato"=FALSE, "In marcia"=FALSE, "Fine rampa V"=FALSE, "Vstabile"=FALSE}}, "DC-REG con eccit."={"Rif Varm"=0.0, "Abilita"=FALSE, "Start\\stop"=FALSE, "Stato"={"Rif Varm"=0.0, "Abilitato"=FALSE, "In marcia"=FALSE, "Fine rampa V"=FALSE, "Vstabile"=FALSE, "PID Varm"=FALSE, "Rif Vecc"=0.0, "PID Vecc"=FALSE}, "Rif Vecc"=0.0}, "AFE (carico elettronico)"={"Rif Id"=0.0, "Abilita"=FALSE, "Start\\stop"=FALSE, "Stato"={"Rif Id"=0.0, "Rif Iq"=0.0, "Abilitato"=FALSE, "In marcia"=FALSE, "Fine rampa Id"=FALSE, "Fine rampa Iq"=FALSE, "Id stabile"=FALSE, "Iq stabile"=FALSE, "PID Id"=FALSE, "PID Iq"=FALSE}, "Rif Iq"=0.0}}  # Comandi alimentatori
        n12 = call <vilib>:"Application Directory.vi"() -> ("Application Directory"=w55:path)
        n13 = Build Path(base path=w55, name or relative path="Settings\\Configurazione_Alimentatori") -> (appended path=w49:path)
        n14 = Open/Create/Replace File(file path (use dialog)=w49, operation (0:open)=T8."open or create") -> (refnum out=w51:refnum<file>, error out=w53:errorcluster)  [unwired: 4 in, 1 out]
        n15 = Read from Binary File(5:T5[] [{"Rif1 max"=400.0, "Rif2 max"=60.0, "Tipo"=enum."ALIMENTATORE AC", "Nome"="", "Controllo Rif 1"={"PID gains"={"proportional gain (Kc)"=0.4, "integral time (Ti, min)"=0.025, "derivative time (Td, min)"=0.0}, "Abilita pid"=FALSE, "Precisione pid"=1.0, "Medie pid"=10, "Trampa[s]"=10, "Tstab ramp[s]"=10, "Max%pid"=10}, "Controllo Rif 2"={"PID gains"={"proportional gain (Kc)"=0.4, "integral time (Ti, min)"=0.025, "derivative time (Td, min)"=0.0}, "Abilita pid"=FALSE, "Precisione pid"=1.0, "Medie pid"=10, "Trampa[s]"=10, "Tstab ramp[s]"=10, "Max%pid"=10}, "note"=""}] ("Array alimentatori"), 8:w53, 11:w51) -> (0:w54:errorcluster, 2:w46:T5[], 3:w52:refnum<file>)  [unwired: 3 in, 1 out]
        n16 = Array Size(array=w46) -> (size(s)=w44:i32)
        n17 = Close File(refnum=w52, error in=w54) -> ()  [unwired: 2 out]
        n18 = local write "Array alimentatori"(w46) -> ()
        n19 = Initialize Array(w61, w44) -> (w60:T2[])
        n20 = Initialize Array(w57, w44) -> (w56:T4)
        n21 = Initialize Array(T7 {"RIF 1"=0.0, "RIF 2"=0.0, "Status"={"Ready"=FALSE, "Running"=FALSE, "Regulation"=FALSE, "Stable"=FALSE}, "Command"={"Start"=FALSE, "Stop"=FALSE}} ("Cluster"), w44) -> (w43:T11)
        n22 = local write "Array pannelli alimentatori"(w56) -> ()
        n23 = Enqueue Element(queue=w59, element=cluster{"Status":string, "variant":variant} {"Status"="REGOLA", "variant"=variant}) -> ()  [unwired: 2 in, 3 out]
      }
      frame "AGGIORNA COMANDI ALIMENTATORE" {
        n24 = Variant To Data(type=T1 {"RIF 1"=0.0, "RIF 2"=0.0, "Status"={"Ready"=FALSE, "Running"=FALSE, "Regulation"=FALSE}, "Start\\stop"={"Start"=FALSE, "Stop"=FALSE}, "PID RIF1"=FALSE, "PID RIF2"=FALSE, "Status ref"={"RIF 1"=0.0, "RIF 2"=0.0}, "Abilita"={"Abilita"=FALSE}} ("Alimentatore 1"), Variant=w84) -> (data=w63:T1)  [unwired: 1 in, 1 out]
        n25 = local write "Alimentatore"(w63) -> ()
        n26 = Index Array(array=w74, index=w64) -> (element=w78:T12)
        n27 = Unbundle By Name(w63) -> ("Abilita.Abilita"=w67:bool, "RIF 1"=w77:dbl, "RIF 2"=w76:dbl, "Start\\stop"=w70:cluster{"Start":bool, "Stop":bool}, "PID RIF1"=w83:bool)  [unwired: 1 out]
        n28 = Bundle By Name(cluster=w78, "RIF1"=w77, "RIF2"=w76, "Command"=w70) -> (w75:T12)
        n29 = Index Array(array=w81, index=w64) -> (element=w82:T5)
        n30 = Bundle By Name(cluster=w82, "Controllo Rif 1.Abilita pid"=w83, "Controllo Rif 2.Abilita pid"=FALSE) -> (w80:T5)
        n31 = Unbundle By Name(w70) -> ("Start"=w69:bool, "Stop"=w68:bool)
        n32 = Replace Array Subset(array=w81, new element=w80, index=w64) -> (w79:T5[])
        n33 = Replace Array Subset(array=w74, new element=w75, index=w64) -> (w73:T9)
        n34 = case shown="True" w69 {
          tunnel: w66 -> [_ w91]
          frame False {
          }
          frame True {
            n35 = Enqueue Element(queue=w91, element=cluster{"Status":string, "variant":variant} {"Status"="START", "variant"=variant}) -> ()  [unwired: 2 in, 3 out]
          }
        }
        n36 = case shown="True" w68 {
          tunnel: w66 -> [_ w89]
          frame False {
          }
          frame True {
            n37 = Enqueue Element(queue=w89, element=cluster{"Status":string, "variant":variant} {"Status"="STOP", "variant"=variant}) -> ()  [unwired: 2 in, 3 out]
          }
        }
        n38 = case shown="True" w67 {
          tunnel: w66 -> [w85 w87]
          frame False {
            n39 = Enqueue Element(queue=w85, element=cluster{"Status":string, "variant":variant} {"Status"="DISABILITA", "variant"=variant}) -> ()  [unwired: 2 in, 3 out]
          }
          frame True {
            n40 = Enqueue Element(queue=w87, element=cluster{"Status":string, "variant":variant} {"Status"="ABILITA", "variant"=variant}) -> ()  [unwired: 2 in, 3 out]
          }
        }
      }
      frame "SELEZIONA ALIMENTATORE" {
        n41 = Variant To Data(type=0, Variant=w100) -> (data=w98:i32)  [unwired: 1 in, 1 out]
      }
      frame "AGGIORNA SETTINGS ALIMENTATORI" {
      }
      frame "REGOLA" {
        w126 = 200
        n42 = Index Array(array=w109, index=w111) -> (element=w110:T5)
        n43 = Wait Until Next ms Multiple(millisecond multiple=w126) -> ()  [unwired: 1 out]
        n44 = Unbundle By Name(w110) -> ("Nome"=→"Nome":string, "Tipo"=w117:T13, "Rif1 max"=w115:dbl, "Rif2 max"=w114:dbl, "Controllo Rif 1"=w116:T14, "Controllo Rif 2"=w113:T14)
        n45 = Enqueue Element(queue=w118, element=cluster{"Status":string, "variant":variant} {"Status"="REGOLA", "variant"=variant}) -> ()  [unwired: 2 in, 3 out]
        n46 = Index Array(array=w124, index=w111) -> (element=w106:T2)
        n47 = case shown="\"VARIAC AC aumenta diminuisci\"" w117 {
          tunnel: w116 -> [w139 w186 w208 w223 _ w256 w270 _]
          tunnel: w115 -> [w166 w202 w218 w239 _ w266 w281 _]
          tunnel: w126 -> [w165 w201 w215 w238 _ w261 w275 _]
          tunnel: w114 -> [w164 w200 _ _ _ _ _ _]
          tunnel: w113 -> [w134 w185 _ _ _ _ _ _]
          tunnel: "Misure" -> [w161 w199 w217 _ w254 w268 w282 _]
          tunnel: w106 -> [w155 w195 w206 w230 w253 w265 w280 w283]
          tunnel: [w160 w198 w213 w236 w252 w264 w279 w283] -> w112
          tunnel: w108 -> [w159 w197 w212 w235 w242 w262 w277 _]
          tunnel: w121 -> [w158 w196 w211 w234 _ w260 w276 _]
          frame "ALIMENTATORE AC", Default {
            w128 = u16 1 items=["Controllo Tensione", "Controllo Frequenza", "Nessun Controllo su WT"] ("Tipo di controllo real time")
            w129 = u16 0 items=["Controllo Tensione", "Controllo Frequenza", "Nessun Controllo su WT"] ("Tipo di controllo real time")
            n48 = global read "Stato alimentatore 1.vi" "Stato alimentatore 1"() -> (w131:T15)
            n49 = Unbundle By Name(w155) -> ("Alimentatore AC.Rif tensione [V]"=w154:dbl, "Alimentatore AC.Rif Freq [Hz]"=w153:dbl)
            n50 = Unbundle By Name(w161) -> ("Vac"=w163:dbl, "F"=w162:dbl)
            n51 = Unbundle By Name(w131) -> ("In marcia"=w130:bool)
            n52 = Not(x=w130) -> (.not. x?=w144:bool)
            n53 = call "Elapsed Time3"("Time Target (s)"=15.0, "Reset"=w144, "Auto Reset"=FALSE) -> ("Time has Elapsed"=w127:bool)  [unwired: 9 in, 7 out]
            n54 = Unbundle By Name(w159) -> ("RIF 1"=w157:dbl, "RIF 2"=w156:dbl)
            n55 = Unbundle By Name(w139) -> ("Abilita pid"=w137:bool)
            n56 = Unbundle By Name(w134) -> ("Abilita pid"=w132:bool)
            n57 = And(x=w127, y=w137) -> (x .and. y?=w136:bool)
            n58 = And(x=w127, y=w132) -> (x .and. y?=w133:bool)
            n59 = Bundle By Name(cluster=w139, "Abilita pid"=w136) -> (w138:T14)
            n60 = Bundle By Name(cluster=w134, "Abilita pid"=w133) -> (w135:T14)
            n61 = Unbundle By Name(w138) -> ("Abilita pid"=w141:bool)
            n62 = Unbundle By Name(w135) -> ("Abilita pid"=w140:bool)
            n63 = call "CONTROLLO RIFERIMENTO.vi"("Controllo"=w135, "SET rampa"=w156, "Lettura reale"=w162, "New value?"=w158, "RIFERIMENTO% in"=w153, "SET pid"=w156, "Valore MAX"=w164, "Tciclo ms"=w165, "Tipo di controllo real time"=w128, "Anche se freno off"=TRUE) -> ("RIFERIMENTO% out"=w152:dbl, "Stabile?"=w147:bool, "fine rampa"=w149:bool)  [unwired: 7 in]
            n64 = call "CONTROLLO RIFERIMENTO.vi"("Controllo"=w138, "SET rampa"=w157, "Lettura reale"=w163, "New value?"=w158, "RIFERIMENTO% in"=w154, "SET pid"=w157, "Valore MAX"=w166, "Tciclo ms"=w165, "Tipo di controllo real time"=w129, "Anche se freno off"=TRUE) -> ("RIFERIMENTO% out"=w151:dbl, "Stabile?"=w148:bool, "fine rampa"=w150:bool)  [unwired: 7 in]
            n65 = Bundle By Name(cluster=w155, "Alimentatore AC.Stato.PID V"=w141, "Alimentatore AC.Stato.PID F"=w140, "Alimentatore AC.Rif tensione [V]"=w151, "Alimentatore AC.Rif Freq [Hz]"=w152, "Alimentatore AC.Stato.Fine rampa V"=w150, "Alimentatore AC.Stato.Fine rampa F"=w149, "Alimentatore AC.Stato.Vstabile"=w148, "Alimentatore AC.Stato.F stabile"=w147) -> (w160:T2)
          }
          frame "Carico elettronico AFE" {
            n66 = Unbundle By Name(w195) -> ("AFE (carico elettronico).Rif Id"=w194:dbl, "AFE (carico elettronico).Rif Iq"=w193:dbl)
            n67 = Unbundle By Name(w199) -> ("Vac"=w170:dbl, "Q"=w178:dbl, "P"=w177:dbl)
            n68 = Unbundle By Name(w197) -> ("RIF 1"=w181:dbl, "RIF 2"=w182:dbl)
            n69 = Absolute Value(x=w178) -> (abs(x)=w176:dbl)
            n70 = Absolute Value(x=w177) -> (abs(x)=w175:dbl)
            n71 = Square Root(x=3.0) -> (sqrt(x)=w168:dbl)
            n72 = Multiply(x=w170, y=w168) -> (x*y=w169:dbl)
            n73 = Multiply(x=w168, y=w170) -> (x*y=w171:dbl)
            n74 = Divide(x=w175, y=w171) -> (x/y=w173:dbl)
            n75 = Divide(x=w176, y=w169) -> (x/y=w172:dbl)
            n76 = call "Calcolo rif carico AFE.vi"("CosFi setpoint"=w182, "kVA setpoint"=w181, "Vac letta"=w170) -> ("LIMITAZIONE"=w167:bool, "iq setpoint [A]"=w179:dbl, "id setpoint [A]"=w180:dbl)  [unwired: 6 in]
            n77 = global write "Fine rampa sinus penta.vi" "LIMITAZIONE AFE"(w167) -> ()
            n78 = call "CONTROLLO RIFERIMENTO.vi"("Controllo"=w186, "SET rampa"=w180, "Lettura reale"=w173, "New value?"=w196, "RIFERIMENTO% in"=w194, "SET pid"=w180, "Valore MAX"=w202, "Tciclo ms"=w201) -> ("RIFERIMENTO% out"=w191:dbl, "Stabile?"=w188:bool, "fine rampa"=w190:bool)  [unwired: 9 in]
            n79 = call "CONTROLLO RIFERIMENTO.vi"("Controllo"=w185, "SET rampa"=w179, "Lettura reale"=w172, "New value?"=w196, "RIFERIMENTO% in"=w193, "SET pid"=w179, "Valore MAX"=w200, "Tciclo ms"=w201) -> ("RIFERIMENTO% out"=w192:dbl, "Stabile?"=w187:bool, "fine rampa"=w189:bool)  [unwired: 9 in]
            n80 = Unbundle By Name(w186) -> ("Abilita pid"=w183:bool)
            n81 = Unbundle By Name(w185) -> ("Abilita pid"=w184:bool)
            n82 = Bundle By Name(cluster=w195, "AFE (carico elettronico).Stato.PID Id"=w183, "AFE (carico elettronico).Stato.PID Iq"=w184, "AFE (carico elettronico).Rif Id"=w191, "AFE (carico elettronico).Rif Iq"=w192, "AFE (carico elettronico).Stato.Fine rampa Id"=w190, "AFE (carico elettronico).Stato.Fine rampa Iq"=w189, "AFE (carico elettronico).Stato.Id stabile"=w188, "AFE (carico elettronico).Stato.Iq stabile"=w187) -> (w198:T2)
          }
          frame "VARIAC AC rif analogico" {
            n83 = Unbundle By Name(w206) -> ("Variac rif analogico.Rif tensione [V]"=w205:dbl)
            n84 = Unbundle By Name(w217) -> ("Vac"=w216:dbl)
            n85 = Unbundle By Name(w212) -> ("RIF 1"=w210:dbl)
            n86 = Unbundle By Name(w208) -> ("Abilita pid"=w207:bool)
            n87 = call "CONTROLLO RIFERIMENTO.vi"("Controllo"=w208, "SET rampa"=w210, "Lettura reale"=w216, "New value?"=w211, "RIFERIMENTO% in"=w205, "SET pid"=w210, "Valore MAX"=w218, "Tciclo ms"=w215) -> ("RIFERIMENTO% out"=w214:dbl, "Stabile?"=w209:bool, "fine rampa"=w203:bool)  [unwired: 9 in]
            n88 = And(x=w209, y=w203) -> (x .and. y?=w204:bool)
            n89 = Bundle By Name(cluster=w206, "Variac rif analogico.Rif tensione [V]"=w214, "Variac rif analogico.Stato.Fine rampa V"=w203, "Variac rif analogico.Stato.Vstabile"=w204, "Variac rif analogico.Stato.PID V"=w207) -> (w213:T2)
          }
          frame "DCREG con eccitazione" {
            # "RIF VARM IN ERALTà è RIF RPM !!!"
            n90 = Unbundle By Name(w223) -> ("Abilita pid"=w225:bool)
            n91 = global read "Fine rampa sinus penta.vi" "Fine Rampa DCREG"() -> (w224:bool)
            n92 = Unbundle By Name(w235) -> ("RIF 1"=w233:dbl, "RIF 2"=w226:dbl)
            n93 = local read "RPM"() -> (w219:dbl)
            n94 = Unbundle By Name(w230) -> ("DC-REG con eccit..Rif Varm"=w229:dbl)
            n95 = And(x=w224, y=w225) -> (x .and. y?=w222:bool)
            n96 = Bundle By Name(cluster=w223, "Abilita pid"=w222) -> (w221:T14)
            n97 = Unbundle By Name(w221) -> ("Abilita pid"=w231:bool)
            n98 = call "CONTROLLO RIFERIMENTO.vi"("Controllo"=w221, "SET rampa"=w233, "Lettura reale"=w219, "New value?"=w234, "RIFERIMENTO% in"=w229, "SET pid"=w233, "Valore MAX"=w239, "Tciclo ms"=w238, "Anche se freno off"=TRUE) -> ("RIFERIMENTO% out"=w237:dbl, "Stabile?"=w232:bool, "fine rampa"=w227:bool)  [unwired: 8 in]
            n99 = And(x=w232, y=w227) -> (x .and. y?=w228:bool)
            n100 = Bundle By Name(cluster=w230, "DC-REG con eccit..Rif Varm"=w237, "DC-REG con eccit..Stato.Fine rampa V"=w227, "DC-REG con eccit..Stato.Fine rampa V"=w228, "Alimentatore AC.Stato.PID V"=w231, "DC-REG con eccit..Rif Vecc"=w226) -> (w236:T2)
          }
          frame "VARIAC AC aumenta diminuisci" {
            w248 = FALSE
            w249 = 5.0  # Precisione V
            n101 = Unbundle By Name(w254) -> ("Vac"=w245:dbl)
            n102 = Unbundle By Name(w242) -> ("RIF 1"=w241:dbl)
            n103 = Add(x=w249, y=w241) -> (x+y=w251:dbl)
            n104 = Subtract(x=w241, y=w249) -> (x-y=w250:dbl)
            n105 = In Range and Coerce(upper limit=w251, x=w245, lower limit=w250) -> (In Range?=w240:bool)  [unwired: 1 out]
            n106 = Greater?(x=w245, y=w241) -> (0:w244:bool)
            n107 = Not(x=w244) -> (.not. x?=w243:bool)
            n108 = Select(t=w248, s=w240, f=w243) -> (s? t:f=w247:bool)
            n109 = Select(t=w248, s=w240, f=w244) -> (s? t:f=w246:bool)
            n110 = Bundle By Name(cluster=w253, "Variac Aumenta diminuisci.Aumenta"=w247, "Variac Aumenta diminuisci.Diminuisci"=w246, "Variac Aumenta diminuisci.Stato.Fine rampa V"=w240) -> (w252:T2)
          }
          frame "ALIMENTATORE DC" {
            n111 = Unbundle By Name(w268) -> ("Vdc"=w267:dbl)
            n112 = Unbundle By Name(w262) -> ("RIF 1"=w259:dbl)
            n113 = Unbundle By Name(w256) -> ("Abilita pid"=w255:bool)
            n114 = call "CONTROLLO RIFERIMENTO.vi"("Controllo"=w256, "SET rampa"=w259, "Lettura reale"=w267, "New value?"=w260, "SET pid"=w259, "Valore MAX"=w266, "Tciclo ms"=w261) -> ("RIFERIMENTO% out"=w263:dbl, "Stabile?"=w258:bool, "fine rampa"=w257:bool)  [unwired: 10 in]
            n115 = Bundle By Name(cluster=w265, "Alimentatore DC.Rif tensione [V]"=w263, "Alimentatore DC.Stato.Fine rampa V"=w257, "Alimentatore DC.Stato.Vstabile"=w258, "Alimentatore DC.Stato.PID V"=w255) -> (w264:T2)
          }
          frame "ALIMENTATORE eccitazione DC" {
            n116 = Unbundle By Name(w282) -> ("Vecc"=w274:dbl)
            n117 = Unbundle By Name(w277) -> ("RIF 1"=w273:dbl)
            n118 = Unbundle By Name(w270) -> ("Abilita pid"=w269:bool)
            n119 = call "CONTROLLO RIFERIMENTO.vi"("Controllo"=w270, "SET rampa"=w273, "Lettura reale"=w274, "New value?"=w276, "SET pid"=w273, "Valore MAX"=w281, "Tciclo ms"=w275) -> ("RIFERIMENTO% out"=w278:dbl, "Stabile?"=w272:bool, "fine rampa"=w271:bool)  [unwired: 10 in]
            n120 = Bundle By Name(cluster=w280, "Alimentatore eccitazione DC.Rif tensione [V]"=w278, "Alimentatore eccitazione DC.Stato.Fine rampa V"=w271, "Alimentatore eccitazione DC.Stato.Vstabile"=w272, "Alimentatore eccitazione DC.Stato.PID V"=w269) -> (w279:T2)
          }
          frame "LINEA ELETTRICA" {
          }
        }
        n121 = Replace Array Subset(array=w124, new element=w112, index=w111) -> (w123:T2[])
      }
      frame "Aggiorna settings alimentatori" {
        n122 = local read "Array alimentatori"() -> (w285:T5[])
        n123 = Variant To Data(type=w285, Variant=w286) -> (data=w284:T5[])  [unwired: 1 in, 1 out]
      }
      frame "SET" {
        n124 = Variant To Data(type=T9 [] ("Array pannelli alimentatori"), Variant=w300) -> (data=w295:T9)  [unwired: 1 in, 1 out]
        n125 = Enqueue Element(queue=w293, element=cluster{"Status":string, "variant":variant} {"Status"="SET DO", "variant"=variant}) -> ()  [unwired: 2 in, 3 out]
      }
      frame "START" {
        w301 = FALSE ("Value")
        n126 = Index Array(array=w308, index=w303) -> (element=w307:T5)
        n127 = Index Array(array=w312, index=w303) -> (element=w306:T2)
        n128 = Unbundle By Name(w307) -> ("Tipo"=w305:T13)
        n129 = case shown="\"ALIMENTATORE AC\", Default" w305 {
          tunnel: w306 -> [w315 w318 w319 w322 w325 w328 w330 w334]
          tunnel: [w314 w317 w319 w321 w324 w327 w329 w333] -> w304
          frame "ALIMENTATORE AC", Default {
            n130 = Bundle By Name(cluster=w315, "Alimentatore AC.Start\\stop"=TRUE) -> (w314:T2)
          }
          frame "VARIAC AC rif analogico" {
            n131 = Bundle By Name(cluster=w318, "Variac rif analogico.Start\\stop"=TRUE ("Alimentatore AC.Start\\stop")) -> (w317:T2)
          }
          frame "VARIAC AC aumenta diminuisci" {
          }
          frame "ALIMENTATORE DC" {
            n132 = Bundle By Name(cluster=w322, "Alimentatore DC.Start\\stop"=TRUE ("Alimentatore DC.Start\\stop")) -> (w321:T2)
          }
          frame "ALIMENTATORE eccitazione DC" {
            n133 = Bundle By Name(cluster=w325, "Alimentatore eccitazione DC.Start\\stop"=TRUE ("Alimentatore DC ecc.Start\\stop")) -> (w324:T2)
          }
          frame "LINEA ELETTRICA" {
            n134 = Bundle By Name(cluster=w328, "Linea elettrica.Start\\stop"=TRUE ("Linea elettrica.Start\\stop")) -> (w327:T2)
          }
          frame "DCREG con eccitazione" {
            n135 = Bundle By Name(cluster=w330, "DC-REG con eccit..Start\\stop"=TRUE) -> (w329:T2)
          }
          frame "Carico elettronico AFE" {
            n136 = Bundle By Name(cluster=w334, "AFE (carico elettronico).Start\\stop"=TRUE ("AFE (carico elettronico).Start\\stop")) -> (w333:T2)
          }
        }
        n137 = Replace Array Subset(array=w312, new element=w304, index=w303) -> (w310:T2[])
        n138 = property on="Start" class="Bool (strict)"("Value"=w301) -> ()  [unwired: 2 in, 2 out]
        n139 = property on="Stop" class="Bool (strict)"("Value"=w301) -> ()  [unwired: 2 in, 2 out]
      }
      frame "STOP" {
        w335 = FALSE ("Value")
        n140 = Index Array(array=w342, index=w337) -> (element=w341:T5)
        n141 = Index Array(array=w346, index=w337) -> (element=w340:T2)
        n142 = Unbundle By Name(w341) -> ("Tipo"=w339:T13)
        n143 = case shown="\"ALIMENTATORE AC\", Default" w339 {
          tunnel: w340 -> [w349 w352 w353 w356 w359 w362 w364 w368]
          tunnel: [w348 w351 w353 w355 w358 w361 w363 w367] -> w338
          frame "ALIMENTATORE AC", Default {
            n144 = Bundle By Name(cluster=w349, "Alimentatore AC.Start\\stop"=FALSE) -> (w348:T2)
          }
          frame "VARIAC AC rif analogico" {
            n145 = Bundle By Name(cluster=w352, "Variac rif analogico.Start\\stop"=FALSE ("Variac rif analogico.Start\\stop")) -> (w351:T2)
          }
          frame "VARIAC AC aumenta diminuisci" {
          }
          frame "ALIMENTATORE DC" {
            n146 = Bundle By Name(cluster=w356, "Alimentatore DC.Start\\stop"=FALSE ("Alimentatore DC.Start\\stop")) -> (w355:T2)
          }
          frame "ALIMENTATORE eccitazione DC" {
            n147 = Bundle By Name(cluster=w359, "Alimentatore eccitazione DC.Start\\stop"=FALSE ("Alimentatore DC ecc.Start\\stop")) -> (w358:T2)
          }
          frame "LINEA ELETTRICA" {
            n148 = Bundle By Name(cluster=w362, "Linea elettrica.Start\\stop"=FALSE ("Linea elettrica.Start\\stop")) -> (w361:T2)
          }
          frame "DCREG con eccitazione" {
            n149 = Bundle By Name(cluster=w364, "DC-REG con eccit..Start\\stop"=FALSE) -> (w363:T2)
          }
          frame "Carico elettronico AFE" {
            n150 = Bundle By Name(cluster=w368, "AFE (carico elettronico).Start\\stop"=FALSE ("AFE (carico elettronico).Start\\stop")) -> (w367:T2)
          }
        }
        n151 = Replace Array Subset(array=w346, new element=w338, index=w337) -> (w344:T2[])
        n152 = property on="Start" class="Bool (strict)"("Value"=w335) -> ()  [unwired: 2 in, 2 out]
        n153 = property on="Stop" class="Bool (strict)"("Value"=w335) -> ()  [unwired: 2 in, 2 out]
      }
      frame "ABILITA" {
        w369 = FALSE ("Value")
        n154 = Index Array(array=w376, index=w371) -> (element=w375:T5)
        n155 = Index Array(array=w380, index=w371) -> (element=w374:T2)
        n156 = Unbundle By Name(w375) -> ("Tipo"=w373:T13)
        n157 = case shown="\"ALIMENTATORE AC\", Default" w373 {
          tunnel: w374 -> [w383 w386 w387 w390 w393 w396 w397 w400]
          tunnel: [w382 w385 w387 w389 w392 w395 w397 w398] -> w372
          frame "ALIMENTATORE AC", Default {
            n158 = Bundle By Name(cluster=w383, "Alimentatore AC.Abilita"=TRUE) -> (w382:T2)
          }
          frame "VARIAC AC rif analogico" {
            n159 = Bundle By Name(cluster=w386, "Variac rif analogico.Abilita"=TRUE) -> (w385:T2)
          }
          frame "VARIAC AC aumenta diminuisci" {
          }
          frame "ALIMENTATORE DC" {
            n160 = Bundle By Name(cluster=w390, "Alimentatore DC.Abilita"=TRUE ("Alimentatore DC.Start\\stop")) -> (w389:T2)
          }
          frame "ALIMENTATORE eccitazione DC" {
            n161 = Bundle By Name(cluster=w393, "Alimentatore eccitazione DC.Abilita"=TRUE ("Alimentatore DC ecc.Start\\stop")) -> (w392:T2)
          }
          frame "LINEA ELETTRICA" {
            n162 = Bundle By Name(cluster=w396, "Linea elettrica.Abilita"=TRUE ("Linea elettrica.Start\\stop")) -> (w395:T2)
          }
          frame "DCREG con eccitazione" {
          }
          frame "Carico elettronico AFE" {
            n163 = Bundle By Name(cluster=w400, "AFE (carico elettronico).Abilita"=TRUE) -> (w398:T2)
          }
        }
        n164 = Replace Array Subset(array=w380, new element=w372, index=w371) -> (w378:T2[])
        n165 = property on="Start" class="Bool (strict)"("Value"=w369) -> ()  [unwired: 2 in, 2 out]
        n166 = property on="Stop" class="Bool (strict)"("Value"=w369) -> ()  [unwired: 2 in, 2 out]
      }
      frame "DISABILITA" {
        w401 = FALSE ("Value")
        n167 = Index Array(array=w408, index=w403) -> (element=w407:T5)
        n168 = Index Array(array=w412, index=w403) -> (element=w406:T2)
        n169 = Unbundle By Name(w407) -> ("Tipo"=w405:T13)
        n170 = case shown="\"ALIMENTATORE AC\", Default" w405 {
          tunnel: w406 -> [w415 w418 w419 w422 w425 w428 w429 w432]
          tunnel: [w414 w417 w419 w421 w424 w427 w429 w431] -> w404
          frame "ALIMENTATORE AC", Default {
            n171 = Bundle By Name(cluster=w415, "Alimentatore AC.Abilita"=FALSE) -> (w414:T2)
          }
          frame "VARIAC AC rif analogico" {
            n172 = Bundle By Name(cluster=w418, "Variac rif analogico.Abilita"=FALSE) -> (w417:T2)
          }
          frame "VARIAC AC aumenta diminuisci" {
          }
          frame "ALIMENTATORE DC" {
            n173 = Bundle By Name(cluster=w422, "Alimentatore DC.Abilita"=FALSE ("Alimentatore DC.Start\\stop")) -> (w421:T2)
          }
          frame "ALIMENTATORE eccitazione DC" {
            n174 = Bundle By Name(cluster=w425, "Alimentatore eccitazione DC.Abilita"=FALSE ("Alimentatore DC ecc.Start\\stop")) -> (w424:T2)
          }
          frame "LINEA ELETTRICA" {
            n175 = Bundle By Name(cluster=w428, "Linea elettrica.Abilita"=FALSE ("Linea elettrica.Start\\stop")) -> (w427:T2)
          }
          frame "DCREG con eccitazione" {
          }
          frame "Carico elettronico AFE" {
            n176 = Bundle By Name(cluster=w432, "AFE (carico elettronico).Abilita"=FALSE) -> (w431:T2)
          }
        }
        n177 = Replace Array Subset(array=w412, new element=w404, index=w403) -> (w410:T2[])
        n178 = property on="Start" class="Bool (strict)"("Value"=w401) -> ()  [unwired: 2 in, 2 out]
        n179 = property on="Stop" class="Bool (strict)"("Value"=w401) -> ()  [unwired: 2 in, 2 out]
      }
      frame "EXIT" {
        w433 = TRUE
        n180 = property on="EXIT" class="Bool (strict)"("Val(Sgnl)"=w433) -> ()  [unwired: 2 in, 2 out]
      }
    }
    "Comandi alimentatori" <- w17
    "EXIT" <- w27
    "Alimentatore 1" <- w20
    "Iteration in Loop 1" <- w21
    "Alimentatore selez" <- w18
  }
  n181 = while {
    stop <- w476 stop-if-true
    # "mappatura comandi"
    n182 = local read "Array alimentatori"() -> (w454:T5[])
    n183 = local read "Comandi alimentatori"() -> (w474:T2[])
    n184 = local read "Alimentatore selez"() -> (w453:i32)
    n185 = global read "Global FINE AVVIO.vi" "Banco manuale"() -> (w446:bool)
    n186 = Wait Until Next ms Multiple(millisecond multiple=u32 100) -> ()  [unwired: 1 out]
    n187 = global read "Global_All_Data.vi" "All Data"() -> (w445:T22)
    n188 = Unbundle By Name(w445) -> ("MISURE NM.U123_media [V]"=w462:string, "MISURE NM.f [Hz]"=w460:string, "MISURE NM.Uarm[V]"=w459:string, "MISURE NM.Uecc[V]"=w458:string, "MISURE ALL.MISURE WT.Q SIGMA"=w443:dbl, "MISURE ALL.MISURE WT.P SIGMA"=w442:dbl, "MISURE NM.n [rpm]"=w440:string)
    n189 = property on="Boolean" class="Bool (strict)"("Visible"=w446) -> ()  [unwired: 2 in, 2 out]
    n190 = local read "Misure"() -> (w463:T3)
    n191 = Index Array(array=w474, index=w453) -> (element=w473:T2)
    n192 = Index Array(array=w454, index=w453) -> (element=w447:T5)
    n193 = call "String To Dbl.vi"("String"=w440) -> ("Numeric"=→"RPM":dbl)  [unwired: 10 in]
    n194 = call "String To Dbl.vi"("String"=w462) -> ("Numeric"=w461:dbl)  [unwired: 10 in]
    n195 = call "String To Dbl.vi"("String"=w460) -> ("Numeric"=w457:dbl)  [unwired: 10 in]
    n196 = call "String To Dbl.vi"("String"=w459) -> ("Numeric"=w456:dbl)  [unwired: 10 in]
    n197 = call "String To Dbl.vi"("String"=w458) -> ("Numeric"=w455:dbl)  [unwired: 10 in]
    n198 = Unbundle By Name(w447) -> ("Tipo"=w452:T13)
    n199 = Bundle By Name(cluster=w463, "Vac"=w461, "F"=w457, "Vdc"=w456, "Vecc"=w455, "Q"=w443, "P"=w442) -> (w441:T3)
    n200 = local write "Misure"(w441) -> ()
    n201 = case shown="1" w453 {
      tunnel: w473 -> [w482 w595 w730 w769]
      tunnel: T15 {"RIF 1"=0.0, "RIF 2"=0.0, "Abilitato"=FALSE, "In marcia"=FALSE, "Fine rampa RIF1"=FALSE, "Fine rampa RIF2"=FALSE, "Vstabile"=FALSE, "F stabile"=FALSE, "PID RIF1"=FALSE, "PID RIF2"=FALSE, "Alimentatore 1"={"RIF 1"=0.0, "RIF 2"=0.0, "Status"={"Ready"=FALSE, "Running"=FALSE, "Regulation"=FALSE}, "Start\\stop"={"Start"=FALSE, "Stop"=FALSE}, "PID RIF1"=FALSE, "PID RIF2"=FALSE, "Status ref"={"RIF 1"=0.0, "RIF 2"=0.0}, "Abilita"={"Abilita"=FALSE}}} ("output cluster") -> [w481 w594 w729 w768]
      tunnel: [w480 w593 w722 w761] -> w468
      tunnel: w452 -> [w479 w592 _ _]
      tunnel: w447 -> [w478 _ _ _]
      tunnel: w445 -> [w477 w591 _ _]
      frame 0, Default {
        n202 = disable-structure shown="Disabled" {
          disable-tunnel: w482 -> [w488 _]
          disable-tunnel: w481 -> [w487 _]
          disable-tunnel: [w486 _] -> w480
          disable-tunnel: w479 -> [w485 _]
          disable-tunnel: w478 -> [w484 _]
          disable-tunnel: w477 -> [w483 _]
          frame Disabled {
            # "BANCO 1 --- SANTERNO"
            # "mappa uscite"
            n203 = case shown="\"ALIMENTATORE AC\", Default" w485 {
              tunnel: w488 -> [w493 w559 _ _ _ _ _ _]
              tunnel: w487 -> [w489 w558 _ _ _ _ _ _]
              tunnel: [w492 w557 _ _ _ _ _ _] -> w486
              tunnel: w484 -> [w491 w556 _ _ _ _ _ _]
              tunnel: w483 -> [w490 _ _ _ _ _ _ _]
              frame "ALIMENTATORE AC", Default {
                # "SINUS PENTA"
                n204 = disable-structure shown="Enabled" {
                  disable-tunnel: w493 -> [w500 w528]
                  disable-tunnel: [w499 w527] -> w492
                  disable-tunnel: w491 -> [w498 _]
                  disable-tunnel: w490 -> [w497 _]
                  disable-tunnel: w489 -> [_ w529]
                  frame Enabled {
                    n205 = Unbundle By Name(w497) -> ("MISURE ALL.STATO PLC 1.USCITE PLC.DO (bit).Marcia FRENO (1s)"=w496:bool)
                    n206 = call "Elapsed Time"("Time Target (s)"=1.0) -> ()  [unwired: 11 in, 8 out]
                    n207 = case shown="True" TRUE {
                      tunnel: w500 -> [_ w505]
                      tunnel: [w501 w504] -> w499
                      tunnel: w498 -> [_ w503]
                      tunnel: w496 -> [_ w502]
                      frame False {
                        n208 = global read "Stato alimentatore 1.vi" "Stato alimentatore 1"() -> (w501:T15)
                      }
                      frame True {
                        n209 = call "Mappa comandi sinus penta.vi"("In marcia?"=w502, "Alimentatore"=w503, "Comandi alimentatori"=w505) -> ("Stato"=w504:T20)  [unwired: 8 in]
                      }
                    }
                  }
                  frame Disabled {
                    n210 = Unbundle By Name(w528) -> ("Alimentatore AC.Rif tensione [V]"=w516:dbl, "Alimentatore AC.Rif Freq [Hz]"=w522:dbl, "Alimentatore AC.Abilita"=w518:bool, "Alimentatore AC.Start\\stop"=w510:bool, "Alimentatore AC.Stato.Fine rampa V"=w535:bool, "Alimentatore AC.Stato.Fine rampa F"=w534:bool, "Alimentatore AC.Stato.Vstabile"=w533:bool, "Alimentatore AC.Stato.F stabile"=w532:bool, "Alimentatore AC.Stato.PID V"=w531:bool, "Alimentatore AC.Stato.PID F"=w530:bool)
                    n211 = global read "Global rapporto trasfo.vi" "Rapporto trasfo"() -> (w515:dbl)
                    n212 = feedback #1() -> (w526:dbl)  [unwired: 1 in]
                    n213 = feedback-in #1(w516) -> ()
                    n214 = Not Equal?(x=w526, y=w516) -> (x != y?=w525:bool)
                    n215 = feedback #2() -> (w523:dbl)  [unwired: 1 in]
                    n216 = feedback-in #2(w522) -> ()
                    n217 = Divide(x=w516, y=w515) -> (x/y=w514:dbl)
                    n218 = Not Equal?(x=w523, y=w522) -> (x != y?=w524:bool)
                    n219 = In Range and Coerce(upper limit=350.0, x=w514, lower limit=0.0) -> (coerced(x)=w513:dbl)  [unwired: 1 out]
                    n220 = case shown="True" w525 {
                      tunnel: w513 -> [_ w552]
                      frame False {
                      }
                      frame True {
                        n221 = Bundle By Name(cluster=T18 {"AO"=enum."RIF V ALIM 1", "Value"=0.0} ("Cluster SET AO"), "Value"=w552) -> (w554:T18)
                        n222 = Build Array(w554) -> (w553:T18[])
                        n223 = call "SET AO.vi"("Cluster SET AO"=w553) -> ()  [unwired: 10 in, 1 out]
                      }
                    }
                    n224 = call "Impulsi START STOP.vi"("Segnale"=w510) -> ("STOP"=w506:bool, "START"=w509:bool)  [unwired: 9 in]
                    n225 = feedback #3() -> (w517:bool)  [unwired: 1 in]
                    n226 = feedback-in #3(w518) -> ()
                    n227 = Not Equal?(x=w518, y=w517) -> (x != y?=w519:bool)
                    n228 = feedback #4() -> (w521:bool)  [unwired: 1 in]
                    n229 = feedback-in #4(w509) -> ()
                    n230 = feedback #5() -> (w507:bool)  [unwired: 1 in]
                    n231 = feedback-in #5(w506) -> ()
                    n232 = Not Equal?(x=w521, y=w509) -> (x != y?=w520:bool)
                    n233 = Not Equal?(x=w507, y=w506) -> (x != y?=w508:bool)
                    n234 = case shown="True" w519 {
                      tunnel: w518 -> [_ w540]
                      frame False {
                      }
                      frame True {
                        n235 = Bundle By Name(cluster=T16 {"DO"=enum."*ABILITA alimentatore 1", "Value"=FALSE} ("Cluster SET DO"), "Value"=w540) -> (w542:T16)
                        n236 = Build Array(w542) -> (w543:T16[])
                        n237 = call "Set DO.vi"("Cluster SET DO"=w543) -> ()  [unwired: 10 in, 1 out]
                      }
                    }
                    n238 = case shown="True" w520 {
                      tunnel: w509 -> [_ w544]
                      frame False {
                      }
                      frame True {
                        n239 = Bundle By Name(cluster=T16 {"DO"=enum."*START alimentatore 1", "Value"=FALSE} ("Cluster SET DO"), "Value"=w544) -> (w546:T16)
                        n240 = Build Array(w546) -> (w547:T16[])
                        n241 = call "Set DO.vi"("Cluster SET DO"=w547) -> ()  [unwired: 10 in, 1 out]
                      }
                    }
                    n242 = case shown="True" w524 {
                      tunnel: w522 -> [_ w548]
                      frame False {
                      }
                      frame True {
                        n243 = Bundle By Name(cluster=T18 {"AO"=enum."RIF F ALIM 1", "Value"=0.0} ("Cluster SET AO"), "Value"=w548) -> (w550:T18)
                        n244 = Build Array(w550) -> (w549:T18[])
                        n245 = call "SET AO.vi"("Cluster SET AO"=w549) -> ()  [unwired: 10 in, 1 out]
                      }
                    }
                    n246 = case shown="True" w508 {
                      tunnel: w506 -> [_ w536]
                      frame False {
                      }
                      frame True {
                        n247 = Bundle By Name(cluster=T16 {"DO"=enum."*STOP alimentatore 1", "Value"=FALSE} ("Cluster SET DO"), "Value"=w536) -> (w538:T16)
                        n248 = Build Array(w538) -> (w539:T16[])
                        n249 = call "Set DO.vi"("Cluster SET DO"=w539) -> ()  [unwired: 10 in, 1 out]
                      }
                    }
                    n250 = Bundle By Name(cluster=w529, "RIF 1"=w516, "RIF 2"=w522, "Abilitato"=w518, "In marcia"=w510, "Fine rampa RIF1"=w535, "Fine rampa RIF2"=w534, "Vstabile"=w533, "F stabile"=w532, "PID RIF1"=w531, "PID RIF2"=w530) -> (w527:T15)
                  }
                }
              }
              frame "VARIAC AC rif analogico" {
                n251 = disable-structure shown="Enabled" {
                  disable-tunnel: w559 -> [w579 _]
                  disable-tunnel: w558 -> [w578 _]
                  disable-tunnel: [w577 _] -> w557
                  disable-tunnel: w556 -> [w573 _]
                  frame Disabled {
                    n252 = Unbundle By Name(w579) -> ("Variac rif analogico.Rif tensione [V]"=w570:dbl, "Variac rif analogico.Start\\stop"=w567:bool, "Variac rif analogico.Abilita"=w562:bool, "Variac rif analogico.Stato.Fine rampa V"=w561:bool, "Variac rif analogico.Stato.Vstabile"=w560:bool, "Variac rif analogico.Stato.PID V"=w575:bool)  [unwired: 1 out]
                    n253 = Unbundle By Name(w573) -> ("Rif1 max"=w569:dbl)
                    n254 = Divide(x=w570, y=w569) -> (x/y=w572:dbl)
                    n255 = Multiply(x=w572, y=100.0) -> (x*y=w564:dbl)
                    n256 = feedback #6() -> (w565:dbl)  [unwired: 1 in]
                    n257 = feedback-in #6(w564) -> ()
                    n258 = Not Equal?(x=w565, y=w564) -> (x != y?=w563:bool)
                    n259 = case shown="True" w563 {
                      tunnel: w564 -> [_ w580]
                      frame False {
                      }
                      frame True {
                        n260 = Bundle By Name(cluster=T18 {"AO"=enum."RIF V ALIM 1", "Value"=0.0} ("Cluster SET AO"), "Value"=w580) -> (w582:T18)
                        n261 = Build Array(w582) -> (w581:T18[])
                        n262 = call "SET AO.vi"("Cluster SET AO"=w581) -> ()  [unwired: 10 in, 1 out]
                      }
                    }
                    n263 = feedback #7() -> (w568:bool)  [unwired: 1 in]
                    n264 = feedback-in #7(w567) -> ()
                    n265 = Not Equal?(x=w568, y=w567) -> (x != y?=w566:bool)
                    n266 = case shown="True" w566 {
                      tunnel: w567 -> [_ w585]
                      tunnel: w562 -> [_ w584]
                      frame False {
                      }
                      frame True {
                        n267 = Bundle By Name(cluster=T16 {"DO"=enum."*ABILITA alimentatore 1", "Value"=FALSE} ("Cluster SET DO"), "Value"=w584) -> (w588:T16)
                        n268 = Bundle By Name(cluster=T16 {"DO"=enum."*START alimentatore 1", "Value"=FALSE} ("Cluster SET DO"), "Value"=w585) -> (w587:T16)
                        n269 = Build Array(w588, w587) -> (w586:T16[])
                        n270 = call "Set DO.vi"("Cluster SET DO"=w586) -> ()  [unwired: 10 in, 1 out]
                      }
                    }
                    n271 = Bundle By Name(cluster=w578, "RIF 1"=w570, "RIF 2"=0.0 ("Rif Freq [Hz]"), "Abilitato"=w562, "In marcia"=w567, "Fine rampa RIF1"=w561, "Fine rampa RIF2"=w561, "Vstabile"=w560, "F stabile"=w560, "PID RIF1"=w575, "PID RIF2"=FALSE ("PID F")) -> (w577:T15)
                  }
                  frame Enabled {
                  }
                }
              }
              frame "VARIAC AC aumenta diminuisci" {
              }
              frame "ALIMENTATORE DC" {
              }
              frame "ALIMENTATORE eccitazione DC" {
              }
              frame "LINEA ELETTRICA" {
              }
              frame "DCREG con eccitazione" {
              }
              frame "Carico elettronico AFE" {
              }
            }
          }
          frame Enabled {
          }
        }
      }
      frame 1 {
        # "BANCO 2 --- KEB"
        n272 = case shown="\"ALIMENTATORE AC\", Default" w592 {
          tunnel: w595 -> [w617 _ _ _ _ _ w675 _]
          tunnel: w594 -> [_ _ _ _ _ _ w674 _]
          tunnel: [w618 _ _ _ _ _ w673 _] -> w593
          tunnel: w591 -> [w599 _ _ _ _ _ w672 _]
          frame "ALIMENTATORE AC", Default {
            # "ALIMENTATORE KEB"
            n273 = Unbundle By Name(w617) -> ("Alimentatore AC.Rif tensione [V]"=w597:dbl, "Alimentatore AC.Rif Freq [Hz]"=w614:dbl, "Alimentatore AC.Abilita"=w627:bool, "Alimentatore AC.Start\\stop"=w626:bool, "Alimentatore AC.Stato.Fine rampa V"=w625:bool, "Alimentatore AC.Stato.Fine rampa F"=w624:bool, "Alimentatore AC.Stato.Vstabile"=w623:bool, "Alimentatore AC.Stato.F stabile"=w622:bool, "Alimentatore AC.Stato.PID V"=w621:bool, "Alimentatore AC.Stato.PID F"=w620:bool)
            n274 = global read "Global dati targa SINUSPENTA.vi" "Inverti senso di rotazione KEB"() -> (w606:bool)
            n275 = Unbundle By Name(w599) -> ("MISURE ALL.STATO PLC 3.Stato DI_PLC.Alimentatore in marcia"=w596:bool)
            n276 = global read "Global rapporto trasfo.vi" "Rapporto trasfo"() -> (w615:dbl)
            n277 = Divide(x=w597, y=w615) -> (x/y=w609:dbl)
            n278 = disable-structure shown="Enabled" {
              disable-tunnel: w614 -> [w648 _]
              disable-tunnel: w609 -> [w647 _]
              disable-tunnel: [w646 _] -> w600
              frame Enabled {
                n279 = Bundle By Name(cluster=cluster{"Hz":dbl, "V":dbl} {"Hz"=0.0, "V"=0.0} ("Value in"), "Hz"=w648, "V"=w647) -> (w649:cluster{"Hz":dbl, "V":dbl})
                n280 = call "RiferimentoTensioneKEB.vi"("Value in"=w649) -> ("Riferimento Tensione"=w646:sgl)  [unwired: 10 in]
              }
              frame Disabled {
              }
            }
            n281 = Select(t=-1.0, s=w606, f=1.0) -> (s? t:f=w607:dbl)
            n282 = call "Da rif freq a rif RPM.vi"("Riferimento Frequenza"=w614) -> ("Riferimento RPM"=w608:dbl)  [unwired: 10 in]
            n283 = disable-structure shown="Enabled" {
              disable-tunnel: [w637 w643] -> w629
              disable-tunnel: [w636 _] -> _
              disable-tunnel: [w635 w639] -> w628
              disable-tunnel: w626 -> [w634 w642]
              disable-tunnel: w596 -> [_ w645]
              disable-tunnel: w596 -> [_ w640]
              frame Disabled {
                n284 = call "Impulsi START STOP.vi"("Segnale"=w634) -> ("STOP"=w635:bool, "START"=w637:bool)  [unwired: 9 in]
                n285 = feedback #8() -> (w633:bool)  [unwired: 1 in]
                n286 = feedback-in #8(w637) -> ()
                n287 = feedback #9() -> (w632:bool)  [unwired: 1 in]
                n288 = feedback-in #9(w635) -> ()
                n289 = Not Equal?(x=w633, y=w637) -> (x != y?=w638:bool)
                n290 = Not Equal?(x=w632, y=w635) -> (x != y?=w636:bool)
              }
              frame Enabled {
                n291 = Not(x=w642) -> (.not. x?=w641:bool)
                n292 = Not(x=w645) -> (.not. x?=w644:bool)
                n293 = And(x=w641, y=w640) -> (x .and. y?=w639:bool)
                n294 = And(x=w642, y=w644) -> (x .and. y?=w643:bool)
              }
            }
            n295 = Greater?(x=w600, y=120.0) -> (0:w611:bool)
            n296 = feedback #10() -> (w630:bool)  [unwired: 1 in]
            n297 = feedback-in #10(w627) -> ()
            n298 = Bundle By Name(cluster=T20 {"Rif tensione [V]"=0.0, "Rif Freq [Hz]"=0.0, "Abilitato"=FALSE, "In marcia"=FALSE, "Fine rampa V"=FALSE, "Fine rampa F"=FALSE, "Vstabile"=FALSE, "F stabile"=FALSE, "PID V"=FALSE, "PID F"=FALSE, "Alimentatore 1"={"RIF 1"=0.0, "RIF 2"=0.0, "Status"={"Ready"=FALSE, "Running"=FALSE, "Regulation"=FALSE}, "Start\\stop"={"Start"=FALSE, "Stop"=FALSE}, "PID RIF1"=FALSE, "PID RIF2"=FALSE, "Status ref"={"RIF 1"=0.0, "RIF 2"=0.0}, "Abilita"={"Abilita"=FALSE}}} ("Stato"), "Rif tensione [V]"=w597, "Rif Freq [Hz]"=w614, "Abilitato"=w627, "In marcia"=w596, "Fine rampa V"=w625, "Fine rampa F"=w624, "Vstabile"=w623, "F stabile"=w622, "PID V"=w621, "PID F"=w620) -> (w618:T20)
            n299 = Multiply(x=w608, y=w607) -> (x*y=w603:dbl)
            n300 = feedback-in #11(w600) -> ()
            n301 = feedback #11() -> (w602:sgl)  [unwired: 1 in]
            n302 = Not Equal?(x=w627, y=w630) -> (x != y?=w631:bool)
            n303 = feedback #12() -> (w616:dbl)  [unwired: 1 in]
            n304 = feedback-in #12(w603) -> ()
            n305 = Not Equal?(x=w602, y=w600) -> (x != y?=w601:bool)
            n306 = Not Equal?(x=w616, y=w603) -> (x != y?=w612:bool)
            n307 = And(x=w601, y=w611) -> (x .and. y?=w610:bool)
            n308 = call "Elapsed Time4"() -> ("Time has Elapsed"=w598:bool)  [unwired: 12 in, 7 out]
            n309 = case shown="True" w610 {
              tunnel: w600 -> [_ w659]
              frame False {
              }
              frame True {
                n310 = Bundle By Name(cluster=T18 {"AO"=enum."RIF V ALIM 2", "Value"=0.0} ("Cluster SET AO"), "Value"=w659) -> (w657:T18)
                n311 = Build Array(w657) -> (w658:T18[])
                n312 = call "SET AO.vi"("Cluster SET AO"=w658) -> ()  [unwired: 10 in, 1 out]
                n313 = call "Set DO.vi"("Cluster SET DO"=T21 [{"DO"=enum."Abilita Scrittura Dati Keb", "Value"=TRUE}]) -> ()  [unwired: 10 in, 1 out]
              }
            }
            n314 = case shown="True" w612 {
              tunnel: w603 -> [_ w651]
              frame False {
              }
              frame True {
                n315 = Bundle By Name(cluster=T18 {"AO"=enum."RIF F ALIM 2", "Value"=0.0} ("Cluster SET AO"), "Value"=w651) -> (w653:T18)
                n316 = Build Array(w653) -> (w654:T18[])
                n317 = call "SET AO.vi"("Cluster SET AO"=w654) -> ()  [unwired: 10 in, 1 out]
              }
            }
            n318 = case shown="True" w631 {
              tunnel: w627 -> [_ w664]
              frame False {
              }
              frame True {
                n319 = Bundle By Name(cluster=T16 {"DO"=enum."*ABILITA alimentatore 2", "Value"=FALSE} ("Cluster SET DO"), "Value"=w664) -> (w666:T16)
                n320 = Build Array(w666) -> (w667:T16[])
                n321 = call "Set DO.vi"("Cluster SET DO"=w667) -> ()  [unwired: 10 in, 1 out]
              }
            }
            n322 = case shown="True" w598 {
              tunnel: w629 -> [_ w668]
              frame False {
              }
              frame True {
                n323 = Bundle By Name(cluster=T16 {"DO"=enum."*START alimentatore 2", "Value"=FALSE} ("Cluster SET DO"), "Value"=w668) -> (w670:T16)
                n324 = Build Array(w670) -> (w671:T16[])
                n325 = call "Set DO.vi"("Cluster SET DO"=w671) -> ()  [unwired: 10 in, 1 out]
              }
            }
            n326 = case shown="True" w598 {
              tunnel: w628 -> [_ w660]
              frame False {
              }
              frame True {
                n327 = Bundle By Name(cluster=T16 {"DO"=enum."*STOP alimentatore 2", "Value"=FALSE} ("Cluster SET DO"), "Value"=w660) -> (w662:T16)
                n328 = Build Array(w662) -> (w663:T16[])
                n329 = call "Set DO.vi"("Cluster SET DO"=w663) -> ()  [unwired: 10 in, 1 out]
              }
            }
          }
          frame "VARIAC AC rif analogico" {
          }
          frame "VARIAC AC aumenta diminuisci" {
          }
          frame "ALIMENTATORE DC" {
          }
          frame "ALIMENTATORE eccitazione DC" {
          }
          frame "LINEA ELETTRICA" {
          }
          frame "DCREG con eccitazione" {
            n330 = disable-structure shown="Disabled" {
              disable-tunnel: w675 -> [w682 _]
              disable-tunnel: w674 -> [w681 _]
              disable-tunnel: [w680 _] -> w673
              disable-tunnel: w672 -> [w679 _]
              frame Disabled {
                n331 = Unbundle By Name(w679) -> ("MISURE ALL.STATO PLC 1.USCITE PLC.DO (bit).Marcia ALIM (1s)"=w678:bool)
                n332 = call "Elapsed Time2"("Time Target (s)"="Time Target (s)") -> ("Time has Elapsed"=w677:bool)  [unwired: 11 in, 7 out]
                n333 = case shown="True" w677 {
                  tunnel: w682 -> [_ w687]
                  tunnel: w681 -> [_ w686]
                  tunnel: [w683 w685] -> w680
                  tunnel: w678 -> [_ w684]
                  frame False {
                    n334 = global read "Stato alimentatore 1.vi" "Stato alimentatore 1"() -> (w683:T15)
                  }
                  frame True {
                    n335 = call "Mappa comandi DCREG.vi"("In marcia"=w684, "Comandi alimentatori"=w687, "output cluster in"=w686) -> ("output cluster out"=w685:T15)  [unwired: 8 in]
                  }
                }
              }
              frame Enabled {
              }
            }
          }
          frame "Carico elettronico AFE" {
          }
        }
      }
      frame 2 {
        w716 = 10000.0 ("y")
        w712 = 570.0  # Inom AFE
        w717 = 10000.0 ("y")
        w721 = 570.0  # Inom AFE
        # "mappa uscite"
        n336 = Unbundle By Name(w730) -> ("AFE (carico elettronico).Rif Id"=w711:dbl, "AFE (carico elettronico).Rif Iq"=w708:dbl, "AFE (carico elettronico).Abilita"=w700:bool, "AFE (carico elettronico).Start\\stop"=w697:bool, "AFE (carico elettronico).Stato.Fine rampa Id"=w728:bool, "AFE (carico elettronico).Stato.Fine rampa Iq"=w727:bool, "AFE (carico elettronico).Stato.Id stabile"=w726:bool, "AFE (carico elettronico).Stato.Iq stabile"=w725:bool, "AFE (carico elettronico).Stato.PID Id"=w724:bool, "AFE (carico elettronico).Stato.PID Iq"=w723:bool)
        n337 = Add(x=w708, y="y 2") -> (x+y=w707:dbl)
        n338 = Add(x=w711, y="y") -> (x+y=w710:dbl)
        n339 = Divide(x=w710, y=w721) -> (x/y=w720:dbl)
        n340 = Divide(x=w707, y=w712) -> (x/y=w713:dbl)
        n341 = Multiply(x=w720, y=w717) -> (x*y=w719:dbl)
        n342 = Multiply(x=w713, y=w716) -> (x*y=w714:dbl)
        n343 = In Range and Coerce(upper limit=w717, x=w719, lower limit=0.0) -> (coerced(x)=w695:dbl)  [unwired: 1 out]
        n344 = In Range and Coerce(upper limit=w716, x=w714, lower limit=0.0) -> (coerced(x)=w690:dbl)  [unwired: 1 out]
        n345 = feedback-in #13(w695) -> ()
        n346 = feedback #13() -> (w704:dbl)  [unwired: 1 in]
        n347 = Not A Number/Path/Refnum?(number/path/refnum=w695) -> (NaN/Path/Refnum?=w694:bool)
        n348 = Not A Number/Path/Refnum?(number/path/refnum=w690) -> (NaN/Path/Refnum?=w691:bool)
        n349 = feedback #14() -> (w698:bool)  [unwired: 1 in]
        n350 = feedback-in #14(w697) -> ()
        n351 = feedback #15() -> (w701:bool)  [unwired: 1 in]
        n352 = feedback-in #15(w700) -> ()
        n353 = feedback #16() -> (w703:dbl)  [unwired: 1 in]
        n354 = feedback-in #16(w690) -> ()
        n355 = Not Equal?(x=w695, y=w704) -> (x != y?=w705:bool)
        n356 = Not(x=w694) -> (.not. x?=w692:bool)
        n357 = Not(x=w691) -> (.not. x?=w688:bool)
        n358 = Not Equal?(x=w697, y=w698) -> (x != y?=w696:bool)
        n359 = Not Equal?(x=w700, y=w701) -> (x != y?=w699:bool)
        n360 = Not Equal?(x=w690, y=w703) -> (x != y?=w702:bool)
        n361 = And(x=w688, y=w702) -> (x .and. y?=w689:bool)
        n362 = And(x=w692, y=w705) -> (x .and. y?=w693:bool)
        n363 = Bundle By Name(cluster=w729, "RIF 1"=w711, "RIF 2"=w708, "Abilitato"=w700, "In marcia"=w697, "Fine rampa RIF1"=w728, "Fine rampa RIF2"=w727, "Vstabile"=w726, "F stabile"=w725, "PID RIF1"=w724, "PID RIF2"=w723) -> (w722:T15)
        n364 = case shown="True" w696 {
          tunnel: w697 -> [_ w733]
          frame False {
          }
          frame True {
            n365 = Bundle By Name(cluster=T16 {"DO"=enum."*START alimentatore 3", "Value"=FALSE} ("Cluster SET DO"), "Value"=w733) -> (w731:T16)
            n366 = Build Array(w731) -> (w732:T16[])
            n367 = call "Set DO.vi"("Cluster SET DO"=w732) -> ()  [unwired: 10 in, 1 out]
          }
        }
        n368 = case shown="True" w699 {
          tunnel: w700 -> [_ w737]
          frame False {
          }
          frame True {
            n369 = Bundle By Name(cluster=T16 {"DO"=enum."*ABILITA alimentatore 3", "Value"=FALSE} ("Cluster SET DO"), "Value"=w737) -> (w736:T16)
            n370 = Build Array(w736) -> (w735:T16[])
            n371 = call "Set DO.vi"("Cluster SET DO"=w735) -> ()  [unwired: 10 in, 1 out]
          }
        }
        n372 = case shown="True" w693 {
          tunnel: w695 -> [_ w743]
          frame False {
          }
          frame True {
            n373 = Bundle By Name(cluster=T18 {"AO"=enum."RIF V ALIM 3", "Value"=0.0} ("Cluster SET AO"), "Value"=w743) -> (w745:T18)
            n374 = Build Array(w745) -> (w744:T18[])
            n375 = call "SET AO.vi"("Cluster SET AO"=w744) -> ()  [unwired: 10 in, 1 out]
          }
        }
        n376 = case shown="True" w689 {
          tunnel: w690 -> [_ w741]
          frame False {
          }
          frame True {
            n377 = Bundle By Name(cluster=T18 {"AO"=enum."RIF F ALIM 3", "Value"=0.0} ("Cluster SET AO"), "Value"=w741) -> (w739:T18)
            n378 = Build Array(w739) -> (w740:T18[])
            n379 = call "SET AO.vi"("Cluster SET AO"=w740) -> ()  [unwired: 10 in, 1 out]
          }
        }
      }
      frame 3 {
        # "mappa uscite"
        n380 = Unbundle By Name(w769) -> ("Alimentatore AC.Rif tensione [V]"=w759:dbl, "Alimentatore AC.Rif Freq [Hz]"=w757:dbl, "Alimentatore AC.Abilita"=w752:bool, "Alimentatore AC.Start\\stop"=w750:bool, "Alimentatore AC.Stato.Fine rampa V"=w767:bool, "Alimentatore AC.Stato.Fine rampa F"=w766:bool, "Alimentatore AC.Stato.Vstabile"=w765:bool, "Alimentatore AC.Stato.F stabile"=w764:bool, "Alimentatore AC.Stato.PID V"=w763:bool, "Alimentatore AC.Stato.PID F"=w762:bool)
        n381 = Bundle By Name(cluster=w768, "RIF 1"=w759, "RIF 2"=w757, "Abilitato"=w752, "In marcia"=w750, "Fine rampa RIF1"=w767, "Fine rampa RIF2"=w766, "Vstabile"=w765, "F stabile"=w764, "PID RIF1"=w763, "PID RIF2"=w762) -> (w761:T15)
        n382 = Bundle By Name(cluster=T18 {"AO"=enum."RIF V ALIM 4", "Value"=0.0} ("Cluster SET AO"), "Value"=w759) -> (w756:T18)
        n383 = Bundle By Name(cluster=T18 {"AO"=enum."RIF F ALIM 4", "Value"=0.0} ("Cluster SET AO"), "Value"=w757) -> (w755:T18)
        n384 = Bundle By Name(cluster=T16 {"DO"=enum."*ABILITA alimentatore 4", "Value"=FALSE} ("Cluster SET DO"), "Value"=w752) -> (w749:T16)
        n385 = Bundle By Name(cluster=T16 {"DO"=enum."*START alimentatore 4", "Value"=FALSE} ("Cluster SET DO"), "Value"=w750) -> (w748:T16)
        n386 = Build Array(w756, w755) -> (w754:T18[])
        n387 = Build Array(w749, w748) -> (w747:T16[])
        n388 = call "SET AO.vi"("Cluster SET AO"=w754) -> ()  [unwired: 10 in, 1 out]
        n389 = call "Set DO.vi"("Cluster SET DO"=w747) -> ()  [unwired: 10 in, 1 out]
      }
    }
    n390 = local read "Alimentatore 1"() -> (w472:T1)
    n391 = Unbundle By Name(w468) -> ("Vstabile"=w450:bool, "Fine rampa RIF1"=w451:bool, "Abilitato"=w467:bool, "In marcia"=w466:bool, "RIF 1"=w465:dbl, "RIF 2"=w464:dbl)
    n392 = Bundle By Name(cluster=w468, "Alimentatore 1"=w472) -> (w471:T15)
    n393 = And(x=w450, y=w451) -> (x .and. y?=w449:bool)
    n394 = Not(x=w449) -> (.not. x?=w448:bool)
    n395 = global write "Stato alimentatore 1.vi" "Stato alimentatore 1"(w471) -> ()
    n396 = local read "Alimentatore"() -> (w470:T1)
    n397 = Bundle By Name(cluster=w470, "Status.Regulation"=w448, "Status.Ready"=w467, "Status.Running"=w466, "Status ref.RIF 1"=w465, "Status ref.RIF 2"=w464) -> (w469:T1)
    n398 = local write "Alimentatore"(w469) -> ()
    n399 = local read "EXIT"() -> (w476:bool)
  }
  n400 = while {
    tunnel: w4 -> [w771]
    stop <- w770 stop-if-true
    n401 = event shown="[3] \"Alimentatore\": Value Change" {
      selector: _ -> [_ _ _ _ _ _ _]
      dyn-events: _ -> [_ _ _ _ _ _ _]
      timeout: _ -> [_ _ _ _ _ _ _]
      tunnel: w771 -> [_ w775 w777 w781 w787 _ w799]
      tunnel: [_ _ _ _ _ _ TRUE] -> w770
      event Timeout {
        n402 = event-data() -> ()  [unwired: 1 in, 3 out]
      }
      event "Array pannelli alimentatori": Value Change {
        n403 = event-data() -> ()  [unwired: 1 in, 6 out]
        n404 = Bundle By Name(cluster=cluster{"Status":string, "variant":variant} {"Status"="SET", "variant"=variant}, "variant"="Array pannelli alimentatori") -> (w773:cluster{"Status":string, "variant":variant})
        n405 = Enqueue Element(queue=w775, element=w773) -> ()  [unwired: 2 in, 3 out]
      }
      event "Array alimentatori": Value Change {
        n406 = event-data() -> ()  [unwired: 1 in, 6 out]
        n407 = local read "Array alimentatori"() -> (w776:T5[])
        n408 = Bundle By Name(cluster=cluster{"Status":string, "variant":variant} {"Status"="Aggiorna settings alimentatori", "variant"=variant}, "variant"=w776) -> (w778:cluster{"Status":string, "variant":variant})
        n409 = Enqueue Element(queue=w777, element=w778) -> ()  [unwired: 2 in, 3 out]
      }
      event Value Change {
        n410 = event-data() -> ()  [unwired: 1 in, 6 out]
        n411 = local read "Alimentatore"() -> (w780:T1)
        n412 = Bundle By Name(cluster=cluster{"Status":string, "variant":variant} {"Status"="AGGIORNA COMANDI ALIMENTATORE", "variant"=variant}, "variant"=w780) -> (w782:cluster{"Status":string, "variant":variant})
        n413 = Enqueue Element(queue=w781, element=w782) -> ()  [unwired: 2 in, 3 out]
      }
      event "SELEZIONA ALIMENTATORE": Value Change {
        n414 = event-data() -> ()  [unwired: 1 in, 6 out]
        n415 = Bundle By Name(cluster=cluster{"Status":string, "variant":variant} {"Status"="SELEZIONA ALIMENTATORE", "variant"=variant}, "variant"="indice alimentatore") -> (w785:cluster{"Status":string, "variant":variant})
        n416 = Enqueue Element(queue=w787, element=w785) -> ()  [unwired: 2 in, 3 out]
      }
      event "Salva alimentatori": Value Change {
        n417 = event-data() -> ()  [unwired: 1 in, 6 out]
        n418 = local read "Array alimentatori"() -> (w788:T5[])
        n419 = call <vilib>:"Application Directory.vi"() -> ("Application Directory"=w791:path)
        n420 = Build Path(base path=w791, name or relative path="Settings\\Configurazione_Alimentatori") -> (appended path=w790:path)
        n421 = Open/Create/Replace File(file path (use dialog)=w790, operation (0:open)=T8."replace or create") -> (refnum out=w795:refnum<file>, error out=w794:errorcluster)  [unwired: 4 in, 1 out]
        n422 = Write to Binary File(file (use dialog)=w795, data=w788, error in=w794) -> (refnum out=w793:refnum<file>, error out=w792:errorcluster)  [unwired: 3 in, 1 out]
        n423 = Close File(refnum=w793, error in=w792) -> ()  [unwired: 2 out]
      }
      event "EXIT": Value Change {
        n424 = event-data() -> ()  [unwired: 1 in, 6 out]
        n425 = Enqueue Element(queue=w799, element=cluster{"Status":string, "variant":variant} {"Status"="EXIT", "variant"=variant}) -> ()  [unwired: 2 in, 3 out]
      }
    }
  }
